vi "XY_plot_gnuplot.vi"(0 "Plot Array":cluster{dbl[], dbl[]}[](array[cluster])=[{[500.0, 500.0, 953.54, 215.0, 270.0, 320.0, 445.0, 525.0, 600.0, 675.0, 750.0, 825.0, 900.0, 960.0, 1010.0, 1060.0], [4.614524, 4.54365, 5.818368, 0.1374656, 0.6662545, 1.465458, 3.619824, 4.848976, 5.887329, 5.940571, 6.152151, 5.717487, 5.600293, 5.40069, 5.154843, 5.121789]}, {[100.0, 150.0, 215.0, 270.0, 320.0, 445.0, 525.0, 600.0, 675.0, 750.0, 825.0, 900.0, 960.0, 1010.0, 1060.0], [0.002314715, -0.00693192, 0.120417, 0.6880509, 1.519176, 3.513709, 5.065183, 6.116033, 6.096773, 5.938465, 5.593788, 5.5597, 5.387002, 5.304077, 4.887903]}] {"?" format="%.2f"; "?" format="%.2f"}, 1 "Job Directory":path=path "/G4_2_HD/Users/paulhayden/Documents/Projects/Westlakes_resolution") -> (2 "Saved Automatically?":bool, 3 "Tex Info String":string="set term epslatex\nset output \"Plot.eps\"\nset xlabel '$Distance~(m)$'\nset ylabel '$DF~(s/m^3)\\times10^6$'\nset samples 1000\nset pointsize 1.00\nset title '$B38~Centreline~Glc$' 0, 0\nset size 0.75,0.9\n\n#set key 450, -2.5833\n unset key\nset label 1 '~~~~~~~~~~~Angle~(deg)~=~0' at -100, -2.58\nset label 2 '~~~~~~~~~~~Height~(m)~=~5' at -100, -3.27\n set xrange [0 : 500] \n# set autoscale x \n set yrange [0.10000 : 7]\n# set autoscale y \n\nplot \"B38_Centreline_Glc.dat\" index 0 using 1:2 axes x1y1 title '$File=B38R~DDD.xls$' with points 1 1, \\\n\"B38_Centreline_Glc.dat\" index 1 using 1:2 axes x1y1 title '$File=B38R~DDD~1.xls$' with points 1 3", 4 "Plot data file":path)   [LabVIEW 2015]
uses:
  Gnuplot_Label.ctl
  gnuplotScriptComponents/gridlines.ctl
  gnuplotScriptComponents/legendAppearance.ctl
  gnuplotScriptComponents/legendProperties.ctl
  gnuplotScriptComponents/alignment.ctl
  gnuplotScriptComponents/at.ctl
  <vilib>/Analysis/baseanly.llb/Mean (DBL).vi
  Results_plotter_Global.vi
  <vilib>/Analysis/NI_AALBase.lvlib
  <vilib>/Analysis/NI_AALPro.lvlib
panel:
  in  "Current Fit Formula":string
  in  "Show Re-Run Gnuplot?":bool
  in  "Tab Control":T1(tab)
  in  "Plot Title":u16(ring) items=["Title String Only", "Stack::", "RunNum::", "WD::(deg)", "EBD::", "Stack:X:(mm ref TTC)", "User:Comments:", "Run:Messages:", "Exclude:Reason:", "X:Rel:(mm)", "Y:Rel:(mm)", "C:minusBG:(ppm)", "C:LatFit:Max(ppm)", "C:LatFit:SigmaY(mm)", "C:LatFit:Yo(mm)", "C:LatData:Max(ppm)", "Uref::(m/s)", "C:incBG:(ppm)", "C:Variance:(ppm^2)", "C:minusBG:(ppm)Err", "C:LatData:Max(ppm)Err", "BG:Conc:(ppm)", "BG:Variance:(ppm^2)", "BG:Conc:(ppm)Err", "FID:Num:", "FID:Calibration:Filename", "X:Trav:(mm)", "Y:Trav:(mm)", "Z (mm)::", "TrackedStack:Yat0deg:(mm)", "TrackedStack:Xat0deg:(mm)", "TrackedStack:Ycurrent:(mm)", "TrackedStack:Xcurrent:(mm)", "T::(C)", "P:Atm:(mbar)", "MFC:Enable:", "MFC24:Read:(%)", "MFC23:Read:(%)", "Date:of:Measurement", "Time:Measurement:Commenced", "Multi Run:Command:Filename", "Multi Run:Start Time:", "Multi Run:Row:Type", "Time:Stamp:(seconds)", "Original:Results:Filename", "Raw:Data:Filename", "EBD:Comments:", "EBD:Xdim:", "EBD:Ydim:", "EBD:Zdim:", "EBD:RunNum:", "EBD:X-Location:", "EBD:Y-Location:", "Number of Measurements"]
  in  "Plot Title":string
  in  "Added labels":i32[](listbox)
  in  "Show Labels?":bool
  in  "Summarise":u16(ring) items=["All Series", "EBD=0L\\times0W\\times0H @  0X, 0Y__Stack X (mm ref TTC)=Show All__", "EBD=80L\\times160W\\times80H @  -80X, 0Y__Stack X (mm ref TTC)=Show All__", "EBD=80L\\times160W\\times80H @  0X, 0Y__Stack X (mm ref TTC)=Show All__", "EBD=90L\\times180W\\times90H @  0X, 0Y__Stack X (mm ref TTC)=Show All__", "EBD=100L\\times200W\\times100H @  -100X, 0Y__Stack X (mm ref TTC)=Show All__"]
  in  "X Log?":bool
  in  "Y Log?":bool
  in  "Ymin Val":dbl
  in  "Ymin":bool=TRUE
  in  "Xmin Val":dbl
  in  "Xmin":bool=TRUE
  in  "Xmax Val":dbl
  in  "Xmax":bool=TRUE
  in  "Ymax Val":dbl
  in  "Ymax":bool=TRUE
  in  "Major Gridlines":T2
  in  "Minor Gridlines":T2
  out "Time format?":bool
  in  "precision":string
  out "Profile offset":dbl
  in  "Offset?":bool
  in  "Mode":T3
  in  "Separation":dbl=1.2
  in  "Fit Line Width":i32=2
  in  "Fit type":T4(ring)
  in  "Put Coeff\nin Results file":bool
  in  "Analysis":T5(ring)
  in  "Wavelength?":bool
  in  "Auto Zp":bool=TRUE
  in  "Fixed Zp":dbl format="%.2f"
  in  "Something about fit..!":bool
  in  "Fit Line Type":i32=2
  in  "Black and white?":bool
  in  "plot error bars?":bool
  in  "Plot style":u16[](array[ring])=[0, 0, 0, 0, 0, 0, 0, 0, 0, 0, 0] items=["points", "lines", "linespoints"]
  in  "Point Size":dbl=1.2 format="%.2f"
  in  "Graph Height":string="0.9"
  in  "Graph width":string="0.75"
  in  "Reverse order":bool
  in  "Appearance":T6
  in  "Show legend?":bool
  in  "Legend Position":u16(ring) items=["LabVIEW calculated", "top left", "top right", "bottom left", "bottom right", "below"]
  in  "Save data analysis file":bool
  out "Path":path
  in  "Filename Max length":i32=28
  out "With legend":i32=580
  out "No Legend":i32=397
  out "No of Series":i32=2
  out "X location":dbl=-100.0
  out "Y location":dbl=-2.583333333333333
  out "Delta y":dbl=0.6900000000000001
  out "Extra range":dbl
  out "Final Title":string="B38 Centreline Glc"
  out "XY Graph":cluster{dbl[], dbl[]}[](graph)=[{[215.0, 270.0, 320.0, 445.0, 500.0, 500.0, 525.0, 600.0, 675.0, 750.0, 825.0, 900.0, 953.54, 960.0, 1010.0, 1060.0], [0.1374656, 0.6662545, 1.465458, 3.619824, 4.614524, 4.54365, 4.848976, 5.887329, 5.940571, 6.152151, 5.717487, 5.600293, 5.818368, 5.40069, 5.154843, 5.121789]}, {[100.0, 150.0, 215.0, 270.0, 320.0, 445.0, 525.0, 600.0, 675.0, 750.0, 825.0, 900.0, 960.0, 1010.0, 1060.0], [0.002314715, -0.00693192, 0.120417, 0.6880509, 1.519176, 3.513709, 5.065183, 6.116033, 6.096773, 5.938465, 5.593788, 5.5597, 5.387002, 5.304077, 4.887903]}]
  # "Scales"
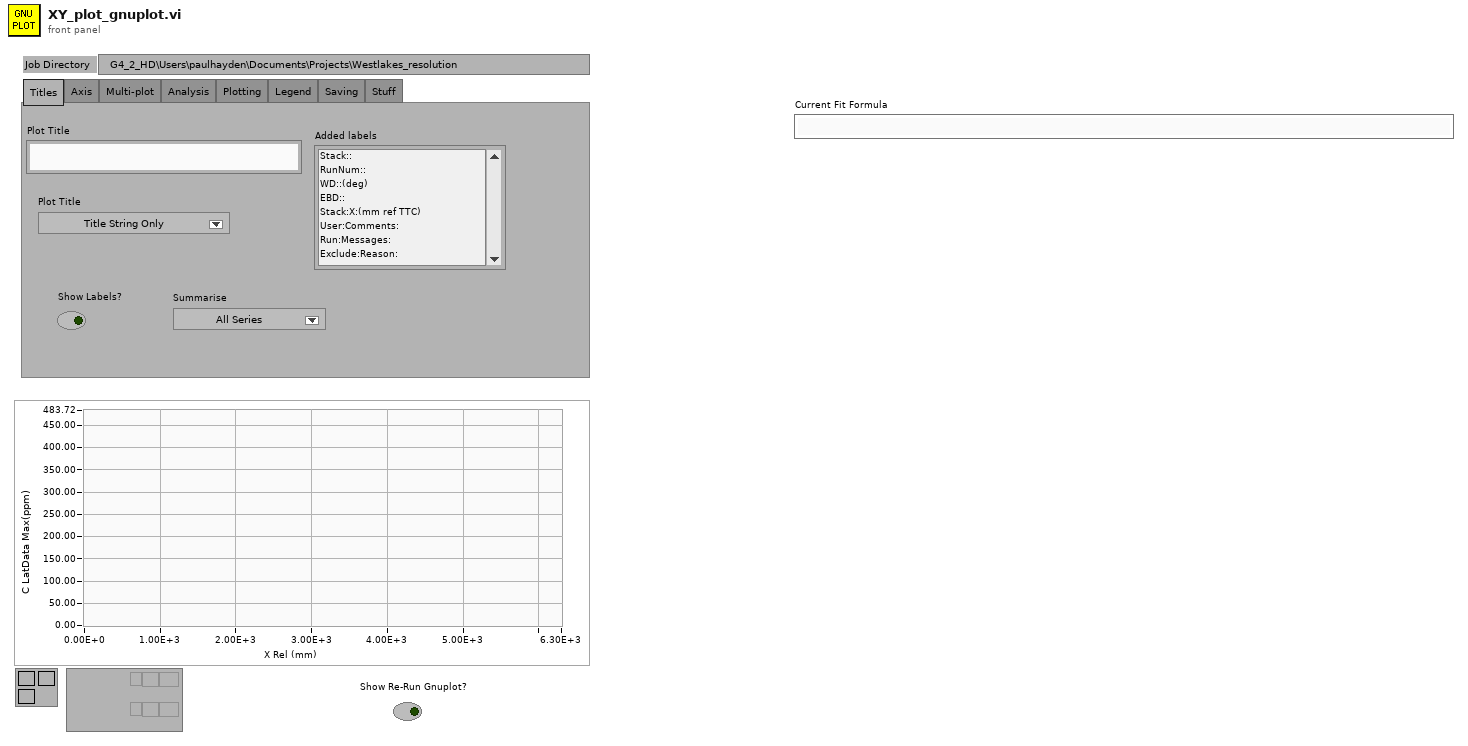
[diagram p1: front panel]
types:
  T1 = enum32{"Titles", "Axis", "Multi-plot", "Analysis", "Plotting", "Legend", "Saving", "Stuff"}
  T2 = typedef "gridlines.ctl" = enum16{"None", "X only", "Y only", "Both X and Y"}
  T3 = typedef "Gnuplot_Label.ctl" = enum16{"3 Labels per plot", "Only Center label", "Only Bottom Label"}
  T4 = enum16{"None", "Spline", "Linear", "2nd Poly", "3rd Poly", "4th Poly", "Gauss Lat", "Gauss vert", "Gauss Vert with 2 sig", "Guass glc"}
  T5 = enum16{"None", "% change", "Spectrum", "Norm Spec"}
  T6 = typedef "legendAppearance.ctl" = cluster{"layout":string, "text-sample order":string, "key order":string, "surroundingBox":string, "MaxRows":u32, "MaxCols":u32, "WidthAdjust":dbl}
  T7 = cluster{"Output":dbl[], "PercentageDifferenceArray":dbl[]}[]
  T8 = cluster{"Output":dbl[], "PercentageDifferenceArray":dbl[]}
  T9 = typedef "legendProperties.ctl" = cluster{"Appearance":T6, "Alignment":T10, "Location":string, "\"At\" location":T11}
  T10 = typedef "alignment.ctl" = cluster{"Horizontal":string, "Vertical":string}
  T11 = typedef "at.ctl" = cluster{"XcoordSys":string, "YcoordSys":string, "Xvalue":dbl, "Yvalue":dbl}
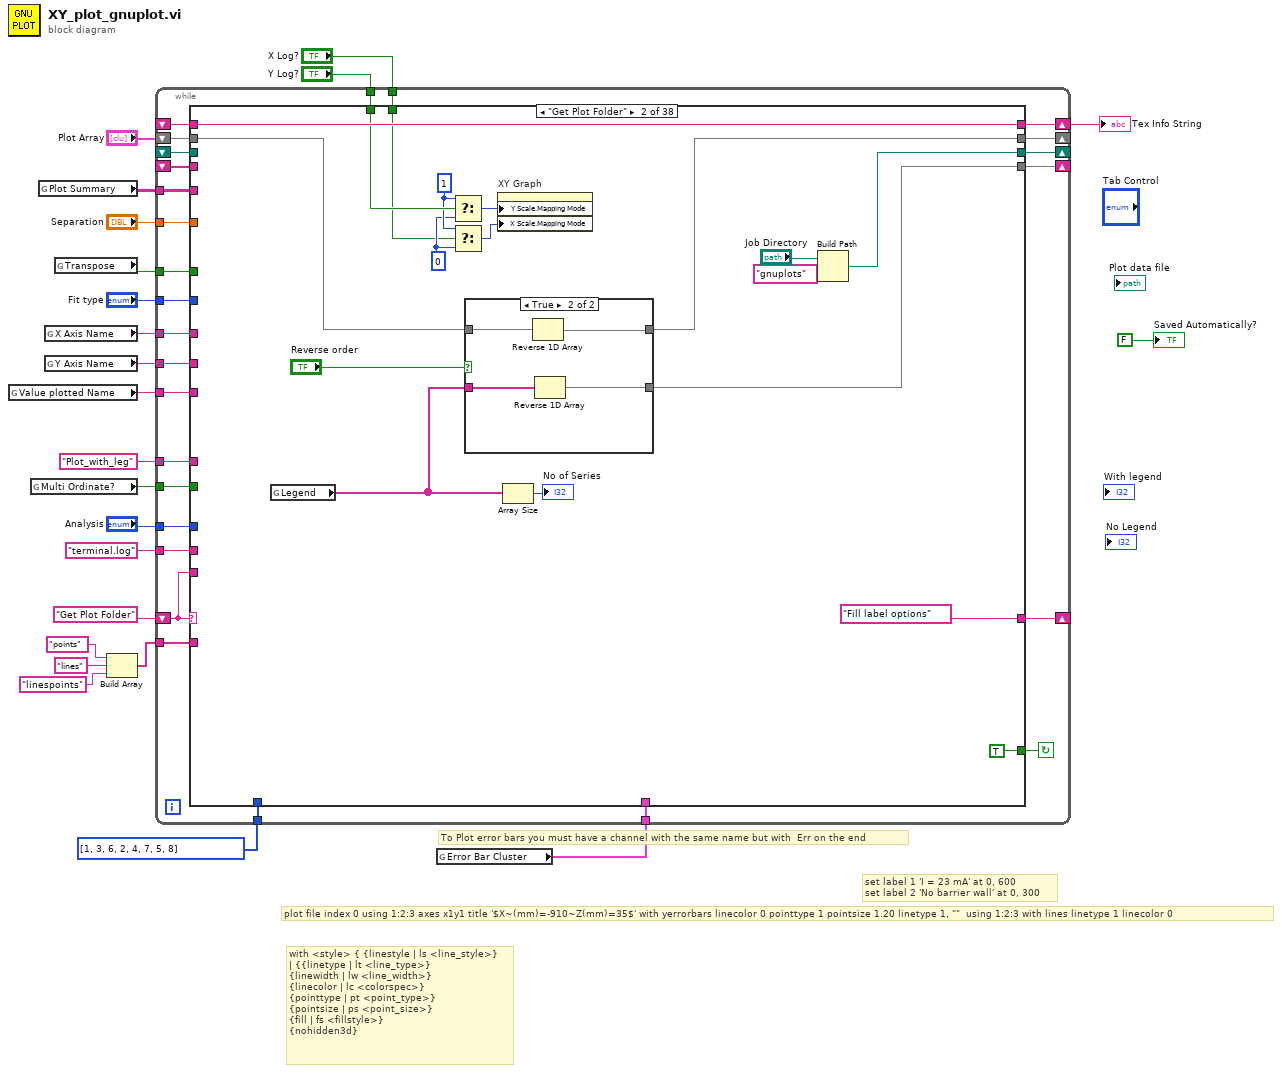
[diagram p0: block diagram]
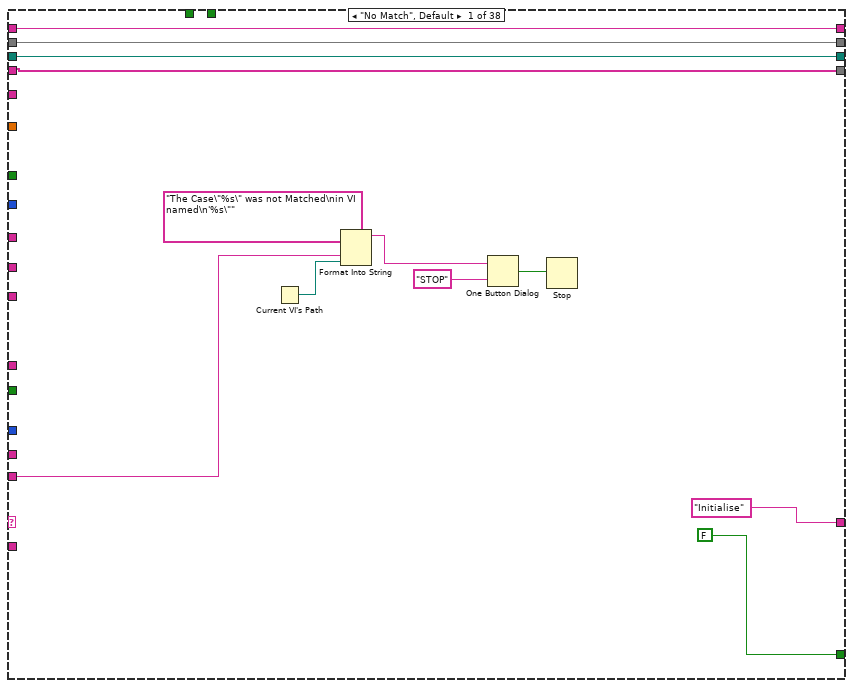
[diagram p2: hidden frame]
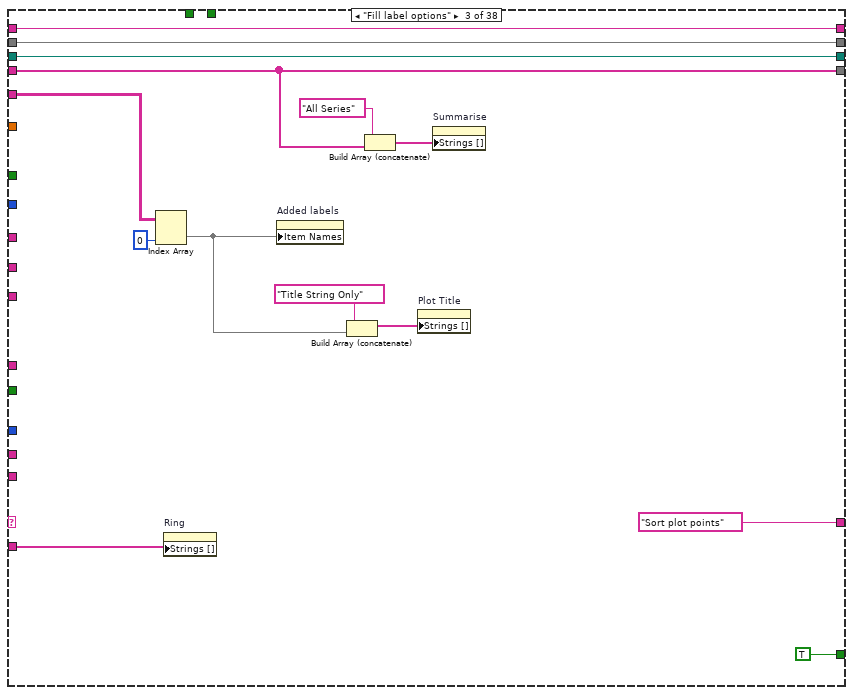
[diagram p4: hidden frame]
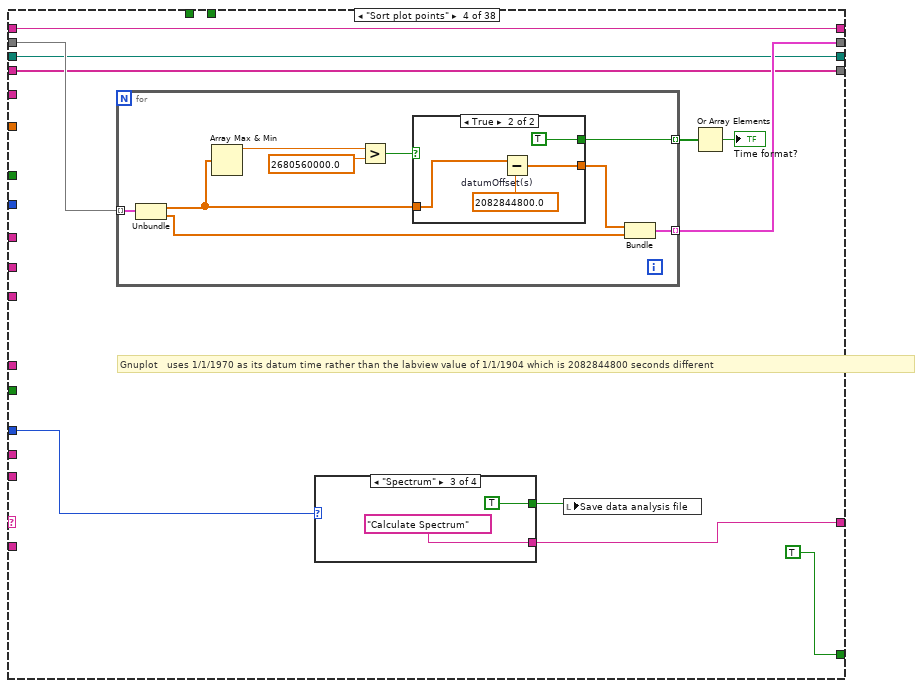
[diagram p5: hidden frame]
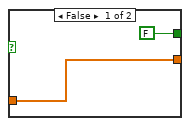
[diagram p6: hidden frame]
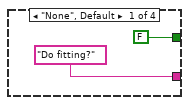
[diagram p7: hidden frame]
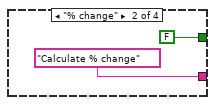
[diagram p8: hidden frame]
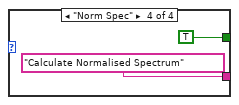
[diagram p9: hidden frame]
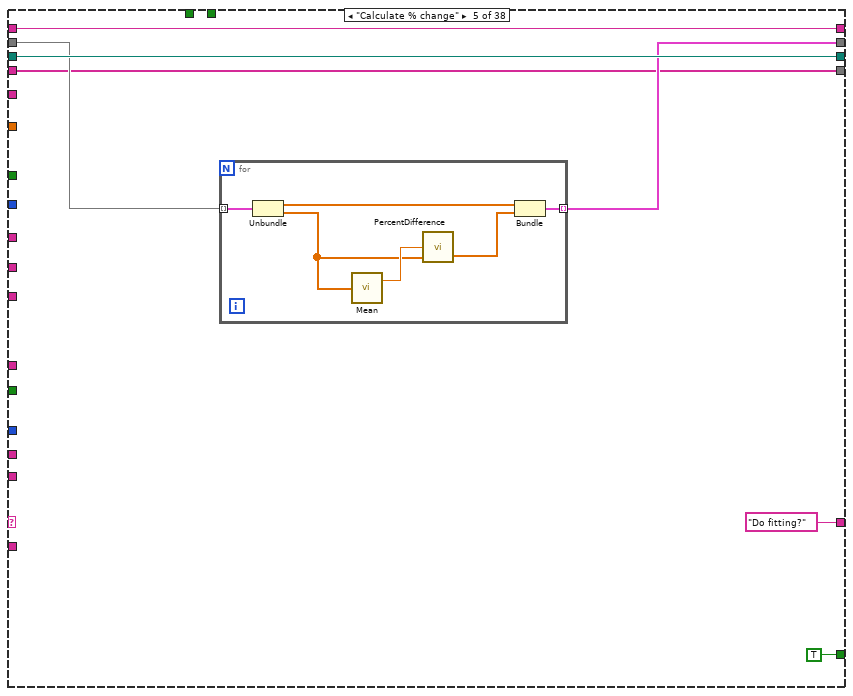
[diagram p10: hidden frame]
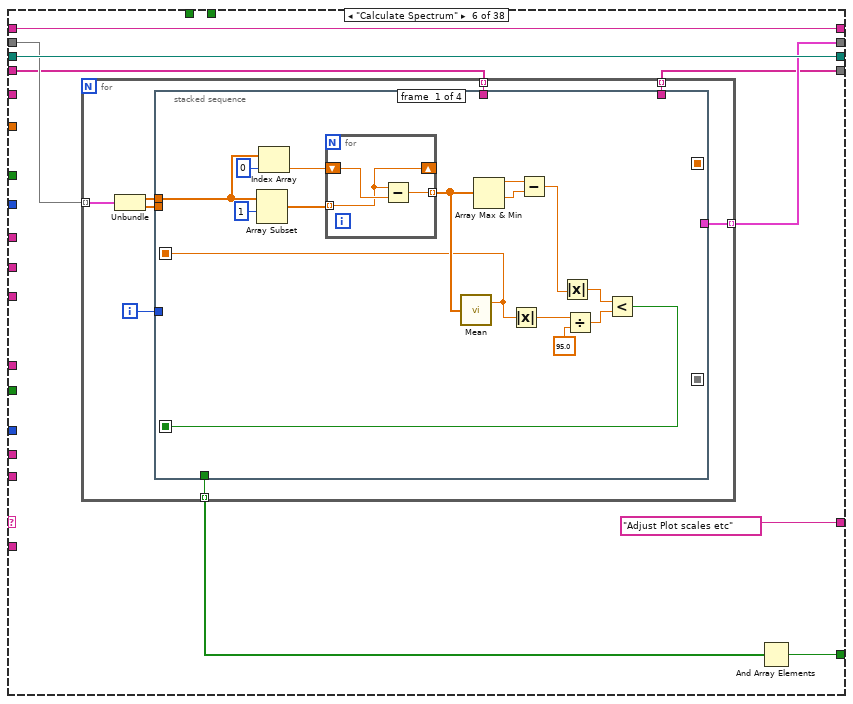
[diagram p11: hidden frame]
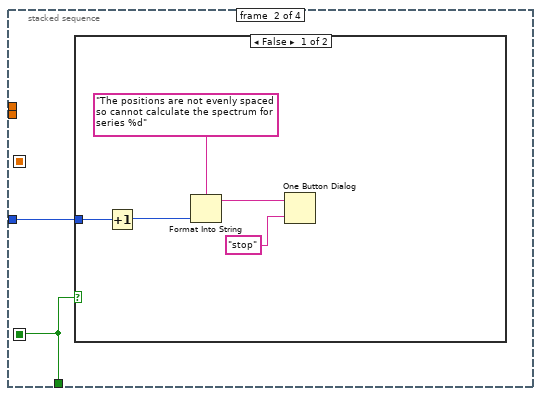
[diagram p12: hidden frame]
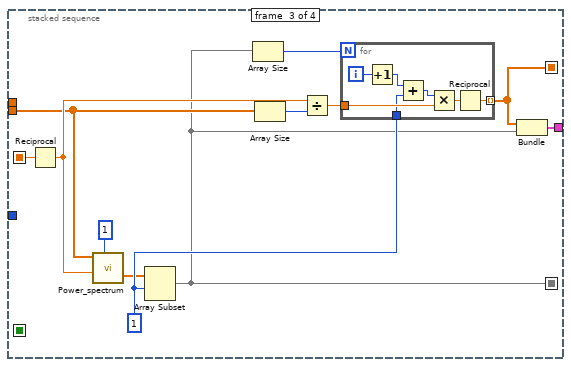
[diagram p14: hidden frame]
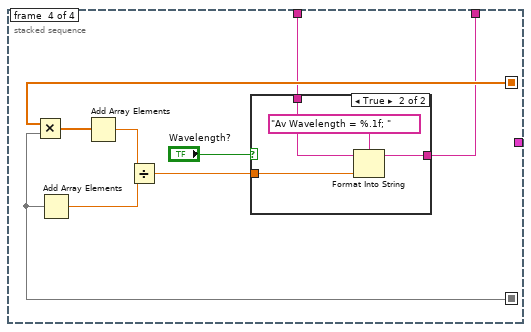
[diagram p15: hidden frame]
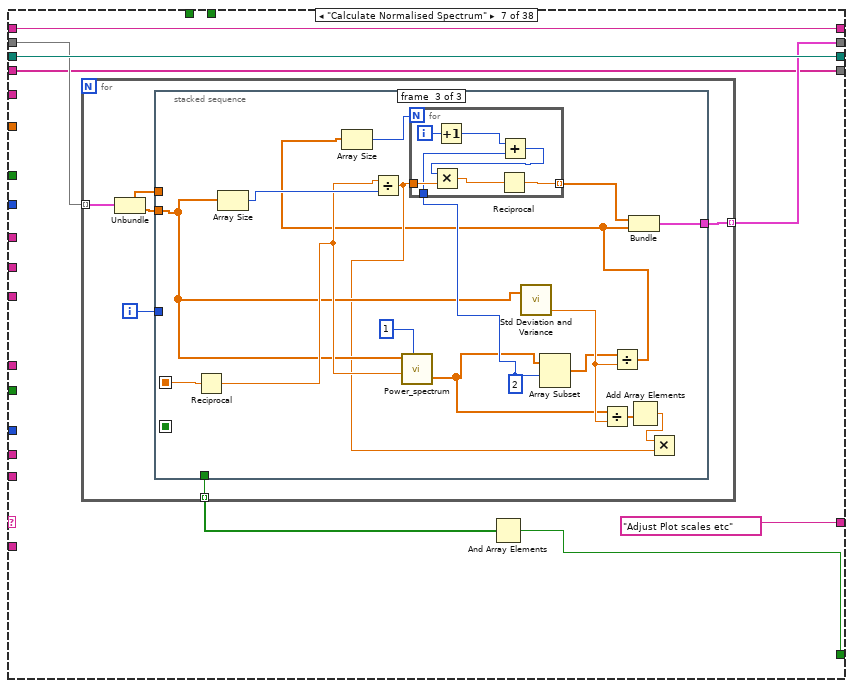
[diagram p17: hidden frame]
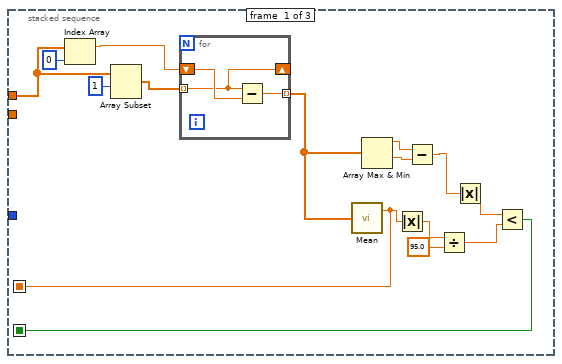
[diagram p18: hidden frame]
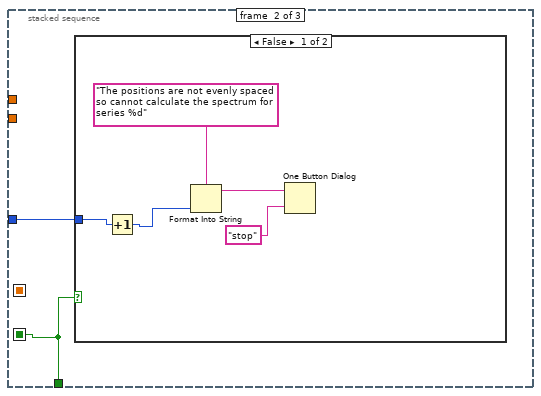
[diagram p19: hidden frame]
diagram:
  # "plot file index 0 using 1:2:3 axes x1y1 title '$X~(mm)=-910~Z(mm)=35$' with yerrorbars linecolor 0 pointtype 1 pointsize 1.20 linetype 1, \"\"  using 1:2:3 with lines linetype 1 linecolor 0"
  # "with <style> { {linestyle | ls <line_style>} \n| {{linetype | lt <line_type>} \n{linewidth | lw <line_width>} \n{linecolor | lc <colorspec>} \n{pointtype | pt <point_type>} \n{pointsize | ps <point_size>} \n{fill | fs <fillstyle>} \n{nohidden3d}"
  # "To Plot error bars you must have a channel with the same name but with  Err on the end"
  # "set label 1 'I = 23 mA' at 0, 600\nset label 2 'No barrier wall' at 0, 300"
  n1 = global read "Results_plotter_Global.vi" "Value plotted Name"() -> (w19:string)
  n2 = global read "Results_plotter_Global.vi" "Multi Ordinate?"() -> (w1:bool)
  n3 = global read "Results_plotter_Global.vi" "Plot Summary"() -> (w22:string[][])
  n4 = global read "Results_plotter_Global.vi" "X Axis Name"() -> (w21:string)
  n5 = global read "Results_plotter_Global.vi" "Y Axis Name"() -> (w20:string)
  n6 = global read "Results_plotter_Global.vi" "Transpose"() -> (w2:bool)
  n7 = Build Array("points", "lines", "linespoints") -> (w9:string[])
  n8 = global read "Results_plotter_Global.vi" "Error Bar Cluster"() -> (w4:cluster{string[]}[])
  n9 = while {
    shift-left: "Get Plot Folder" -> [w48]
    shift-right: [w49] -> _
    tunnel: w22 -> [w47]
    shift-right: [w46] -> _
    shift-left: _ -> [w45]
    tunnel: "Analysis" -> [w44]
    tunnel: w21 -> [w43]
    tunnel: w20 -> [w42]
    tunnel: w19 -> [w41]
    shift-right: [w39] -> _
    shift-left: "Plot Array" -> [w40]
    shift-right: [w37] -> w17
    shift-left: _ -> [w38]
    tunnel: "Plot_with_leg" ("name or relative path") -> [w36]
    tunnel: "Fit type" -> [w35]
    shift-right: [w34] -> _
    shift-left: _ -> [w33]
    tunnel: "terminal.log" -> [w32]
    tunnel: w9 -> [w31]
    tunnel: i32[] [1, 3, 6, 2, 4, 7, 5, 8] ("Plot style") -> [w30]
    tunnel: "Separation" -> [w29]
    tunnel: "Y Log?" -> [w28]
    tunnel: w4 -> [w27]
    tunnel: "X Log?" -> [w26]
    tunnel: w2 -> [w25]
    tunnel: w1 -> [w24]
    stop <- w50 continue-if-true
    n10 = case shown="\"Get Plot Folder\"" w48 {
      tunnel: [FALSE TRUE TRUE ("Top Level") TRUE TRUE w150 w223 TRUE TRUE TRUE ("Top Level") TRUE ("Top Level") TRUE ("Top Level") TRUE ("Top Level") TRUE ("Top Level") TRUE ("Top Level") TRUE ("Top Level") TRUE ("Top Level") TRUE ("Top Level") TRUE ("Top Level") TRUE ("Top Level") w674 w747 TRUE ("Top Level") TRUE ("Top Level") TRUE ("Top Level") TRUE ("Top Level") TRUE ("Top Level") TRUE ("Top Level") TRUE ("Top Level") TRUE ("Top Level") TRUE ("Top Level") TRUE ("Top Level") TRUE ("Top Level") TRUE ("Top Level") TRUE ("Top Level") w1578 FALSE ("Top Level") FALSE ("Top Level")] -> w50
      tunnel: ["Initialise" "Fill label options" "Sort plot points" w104 "Do fitting?" "Adjust Plot scales etc" "Adjust Plot scales etc" "Adjust Plot scales etc" "Add fitted line styles" "Adjust Plot scales etc" w381 "Fill Second legend" "Fill Second legend" "Fill Second legend" "Calculate plot max and min values" "Sort out plot title" w566 w636 "Create plot directory" w660 w673 w746 w890 "Edit Legend names" w1078 "Labels?" ("t") "Labels?" ("t") w1241 w1252 "Plot Command" "Write gnuplot file" ("t") "Execute shell script" ("t") "Has pdf been generated?" ("t") w1554 "Input Fit Coefficients into results file?" "Read Fit Coefficients" ("t") "End" ("t") "End" ("t")] -> w49
      tunnel: w48 -> [w57 _ _ _ _ _ _ _ _ _ _ _ _ _ _ _ _ _ _ _ _ _ _ _ _ _ _ _ _ _ _ _ _ _ _ _ _ _]
      tunnel: w47 -> [_ _ w100 _ _ _ _ _ _ _ _ _ _ _ _ _ w575 _ _ _ w672 w745 _ _ _ _ _ _ w1251 _ _ _ _ _ _ _ _ _]
      tunnel: [w54 w77 w94 w108 w139 w155 w229 w290 w305 w366 w391 w417 w426 w438 w465 w499 w568 w637 w648 w662 w675 w748 w902 w944 w1093 w1161 w1218 w1248 w1258 w1384 w1416 w1539 w1547 w1560 w1571 w1582 w1600 w1727] -> w46
      tunnel: w45 -> [w54 _ w94 w108 w139 w155 w229 w290 w305 w366 w391 w417 w426 w438 w461 w499 w567 w633 w649 w657 w675 w748 w902 w944 w1093 w1161 w1218 w1248 w1258 w1384 w1416 w1539 w1547 w1560 w1571 w1582 w1600 w1727]
      tunnel: w44 -> [_ _ _ w105 _ _ _ _ _ _ w382 _ _ w432 _ _ _ w624 _ _ w668 w740 w899 _ _ _ _ _ _ _ _ _ _ _ _ _ _ _]
      tunnel: w43 -> [_ _ _ _ _ _ _ _ w296 _ _ w413 w425 _ _ _ _ _ _ _ w671 w744 w897 _ _ _ _ _ _ _ _ _ _ _ _ _ _ _]
      tunnel: w42 -> [_ _ _ _ _ _ _ _ w295 _ _ w412 w424 w437 _ _ _ _ _ _ w670 w743 w898 _ _ _ _ _ _ _ _ _ _ _ _ _ _ _]
      tunnel: w41 -> [_ _ _ _ _ _ _ _ _ _ _ _ _ _ _ _ _ _ _ _ w667 _ _ _ _ _ _ _ _ _ _ _ _ _ _ _ w1588 _]
      tunnel: w40 -> [w53 w72 w95 w110 w138 w154 w228 w286 w301 w365 w380 w416 w423 w436 w464 w496 w581 w635 w652 w665 w666 w742 w903 w932 w1088 w1156 w1214 w1245 w1253 w1385 w1417 w1545 w1552 w1567 w1576 w1586 w1593 w1732]
      tunnel: [w53 w71 w95 w109 w137 w153 w227 w286 w294 w365 w380 w416 w423 w436 w464 w496 w581 w635 w652 w665 w666 w739 w903 w932 w1088 w1156 w1214 w1245 w1253 w1385 w1417 w1545 w1552 w1567 w1576 w1586 w1593 w1732] -> w39
      tunnel: w38 -> [w52 w76 w96 w107 w136 w152 w226 w289 w304 w363 w383 w415 w422 w435 w463 w500 w576 w634 w651 w664 w676 w749 _ w942 w1092 w1127 w1194 w1236 w1255 w1382 w1414 w1534 w1550 w1565 w1574 w1584 w1603 w1730]
      tunnel: [w52 w76 w96 w107 w136 w152 w226 w289 w304 w363 w383 w415 w422 w435 w463 w500 w576 w634 w651 w664 w676 w749 w893 w940 w1092 w1124 w1193 w1235 w1256 w1378 w1413 w1534 w1550 w1565 w1574 w1584 w1603 w1730] -> w37
      tunnel: w36 -> [_ _ _ _ _ _ _ _ _ _ _ _ _ _ _ _ _ _ _ _ _ _ _ _ _ _ _ _ _ _ _ _ _ _ _ _ _ _]
      tunnel: w35 -> [_ _ _ _ _ _ _ w287 w303 _ w385 _ _ _ _ _ _ _ _ _ _ _ w891 w946 _ _ _ _ _ w1351 w1410 _ _ _ _ w1581 w1596 _]
      tunnel: [w51 w70 w92 w106 w135 w148 w225 w288 w298 w362 w387 w414 w421 w434 w462 w498 w580 w632 w650 w663 w669 w741 w901 w947 w1094 w1160 w1217 w1247 w1257 w1372 w1415 w1540 w1551 w1566 w1575 w1585 w1604 w1731] -> w34
      tunnel: w33 -> [w51 _ w92 w106 w135 w149 w225 w288 w299 w362 w387 w414 w421 w434 w462 w498 w580 w632 w650 w663 w669 w741 w901 w947 w1095 w1160 w1217 w1247 w1257 w1372 w1415 w1540 w1551 w1566 w1575 w1585 w1604 w1731]
      tunnel: w32 -> [_ _ _ _ _ _ _ _ _ _ _ _ _ _ _ _ _ _ _ _ _ _ _ _ _ _ _ _ _ _ _ _ w1546 _ _ _ _ w1725]
      tunnel: w31 -> [_ _ w90 _ _ _ _ _ _ _ _ _ _ _ _ _ _ _ _ _ _ _ _ _ _ _ _ _ _ _ _ _ _ _ _ _ _ _]
      tunnel: w30 -> [_ _ _ _ _ _ _ _ _ _ _ _ _ _ _ _ _ _ _ _ _ _ _ _ _ _ _ _ _ _ w1408 w1536 _ _ _ _ _ _]
      tunnel: w29 -> [_ _ _ _ _ _ _ _ _ _ _ _ _ _ _ _ _ _ _ _ _ w738 _ _ w1087 _ _ _ _ w1369 _ _ _ _ _ _ _ _]
      tunnel: w28 -> [_ w69 _ _ _ _ _ _ _ _ _ _ _ _ _ _ _ _ _ _ _ _ _ _ _ w1140 w1205 _ w1250 w1366 _ _ _ _ _ _ _ _]
      tunnel: w27 -> [_ _ _ _ _ _ _ _ _ _ _ _ _ _ _ w469 _ _ _ _ _ w737 _ _ _ _ _ _ _ _ w1407 _ _ _ _ _ _ _]
      tunnel: w26 -> [_ w64 _ _ _ _ _ _ _ _ _ _ _ _ _ _ _ _ _ _ _ _ _ _ _ w1137 _ _ w1249 w1361 _ _ _ _ _ _ _ _]
      tunnel: w25 -> [_ _ _ _ _ _ _ _ _ _ _ _ _ _ _ w467 _ _ _ _ _ w736 _ w933 _ _ _ _ _ w1356 w1404 _ _ _ _ _ _ _]
      tunnel: w24 -> [_ _ _ _ _ _ _ _ _ _ _ _ _ _ _ _ _ _ _ _ _ _ _ _ _ _ _ _ _ _ _ _ _ _ _ _ _ _]
      frame "No Match", Default {
        n11 = Current VI's Path() -> (path=w56:path)
        n12 = Format Into String(format string="The Case\"%s\" was not Matched\nin VI named\n'%s\"" ("Format String"), w57, w56) -> (resulting string=w60:string)  [unwired: 2 in, 1 out]
        n13 = One Button Dialog(message=w60, button name ("OK")="STOP") -> (true=w58:bool)
        n14 = Stop(stop? (T)=w58) -> ()
      }
      frame "Get Plot Folder" {
        w65 = u8 0 ("f")
        w66 = u8 1 ("Y Scale.Mapping Mode")
        n15 = global read "Results_plotter_Global.vi" "Legend"() -> (w63:string[])
        n16 = Select(t=w66, s=w69, f=w65) -> (s? t:f=w68:u8)
        n17 = Select(t=w66, s=w64, f=w65) -> (s? t:f=w67:u8)
        n18 = case shown="True" "Reverse order" {
          tunnel: w72 -> [w82 w86]
          tunnel: [w82 w85] -> w71
          tunnel: w63 -> [w81 w84]
          tunnel: [w81 w83] -> w70
          frame False {
          }
          frame True {
            n19 = Reverse 1D Array(array=w86) -> (reversed array=w85:T7)
            n20 = Reverse 1D Array(array=w84) -> (reversed array=w83:string[])
          }
        }
        n21 = property on="XY Graph" class="XYGraph (strict)"("Y Scale.Mapping Mode"=w68, "X Scale.Mapping Mode"=w67) -> ()  [unwired: 2 in, 2 out]
        n22 = Array Size(array=w63) -> (size(s)=→"No of Series":i32)
        n23 = Build Path(base path="Job Directory", name or relative path="gnuplots") -> (appended path=w77:path)
      }
      frame "Fill label options" {
        n24 = Index Array(array=w100, index (col)=0 ("disabled index (col)")) -> (element=w88:string[])  [unwired: 1 in]
        n25 = property on="Ring" class="Ring (strict)"("Strings []"=w90) -> ()  [unwired: 2 in, 2 out]
        n26 = property on="Added labels" class="LstBox (strict)"("Item Names"=w88) -> ()  [unwired: 2 in, 2 out]
        n27 = Build Array (concatenate)("Title String Only", w88) -> (w87:string[])
        n28 = Build Array (concatenate)("All Series", w92) -> (w93:string[])
        n29 = property on="Plot Title" class="Ring (strict)"("Strings []"=w87) -> ()  [unwired: 2 in, 2 out]
        n30 = property on="Summarise" class="Ring (strict)"("Strings []"=w93) -> ()  [unwired: 2 in, 2 out]
      }
      frame "Sort plot points" {
        # "Gnuplot   uses 1/1/1970 as its datum time rather than the labview value of 1/1/1904 which is 2082844800 seconds different"
        n31 = for {
          tunnel: w110 -> [w119] mode=indexing
          tunnel: [w120] -> w109 mode=indexing
          tunnel: [w112] -> w102 mode=indexing
          n32 = Unbundle(w119) -> ("Output"=w115:dbl[], "PercentageDifferenceArray"=w116:dbl[])
          n33 = Array Max & Min(array=w115) -> (max value=w118:dbl)  [unwired: 3 out]
          n34 = Greater?(x=w118, y=2680560000.0) -> (0:w113:bool)
          n35 = case shown="True" w113 {
            tunnel: w115 -> [w122 w126]
            tunnel: [w122 w124] -> w114
            tunnel: [FALSE TRUE] -> w112
            frame False {
            }
            frame True {
              w125 = 2082844800.0  # datumOffset(s)
              n36 = Subtract(x=w126, y=w125) -> (x-y=w124:dbl[])
            }
          }
          n37 = Bundle("Output"=w114, "PercentageDifferenceArray"=w116) -> (w120:T8)  [unwired: 1 out]
        }
        n38 = case shown="\"Spectrum\"" w105 {
          tunnel: ["Do fitting?" "Calculate % change" "Calculate Spectrum" "Calculate Normalised Spectrum"] -> w104
          tunnel: [FALSE ("Save data analysis file") FALSE ("Save data analysis file") TRUE ("Save data analysis file") TRUE ("Save data analysis file")] -> w103
          frame "None", Default {
          }
          frame "% change" {
          }
          frame "Spectrum" {
          }
          frame "Norm Spec" {
          }
        }
        n39 = local write "Save data analysis file"(w103) -> ()
        n40 = Or Array Elements(Boolean array=w102) -> (logical OR=→"Time format?":bool)
      }
      frame "Calculate % change" {
        n41 = for {
          tunnel: w138 -> [w147] mode=indexing
          tunnel: [w145] -> w137 mode=indexing
          n42 = Unbundle(w147) -> ("Output"=w146:dbl[], "PercentageDifferenceArray"=w143:dbl[])
          n43 = call-poly <vilib>:"Mean.vi"("X"=w143) -> ("mean"=w144:dbl)  [unwired: 1 out]
          n44 = call "PercentDifference.vi"("CompareeArray"=w143, "Basis"=w144) -> ("PercentageDifferenceArray"=w142:dbl[])  [unwired: 1 in, 1 out]
          n45 = Bundle("Output"=w146, "PercentageDifferenceArray"=w142) -> (w145:T8)  [unwired: 1 out]
        }
      }
      frame "Calculate Spectrum" {
        n46 = for {
          tunnel: w154 -> [w163] mode=indexing
          tunnel: [w164] -> w153 mode=indexing
          tunnel: [w159] -> w151 mode=indexing
          tunnel: w149 -> [w158] mode=indexing
          tunnel: [w157] -> w148 mode=indexing
          i -> [w160]
          n47 = Unbundle(w163) -> ("Output"=w161:dbl[], "PercentageDifferenceArray"=w162:dbl[])
          n48 = stacked-sequence {
            seq-local: [w166 _ _ _] -> [_ _ w196 _]
            seq-local: [w165 _ _ _] -> [_ w183 _ _]
            seq-local: [_ _ w191 _] -> [_ _ _ w216]
            seq-local: [_ _ w190 _] -> [_ _ _ w217]
            tunnel: [_ _ w201 _] -> w164
            tunnel: w162 -> [_ _ w194 _]
            tunnel: w161 -> [w177 _ _ _]
            tunnel: w160 -> [_ w184 _ _]
            tunnel: [_ w183 _ _] -> w159
            tunnel: w158 -> [_ _ _ w212]
            tunnel: [_ _ _ w210] -> w157
            frame #0 {
              n49 = Array Subset(array=w177, index=1) -> (w175:dbl[])  [unwired: 1 in]
              n50 = Index Array(array=w177, index=0) -> (element=w176:dbl)
              n51 = for {
                shift-right: [w181] -> _
                shift-left: w176 -> [w182]
                tunnel: w175 -> [w181] mode=indexing
                tunnel: [w180] -> w172 mode=indexing
                n52 = Subtract(x=w181, y=w182) -> (x-y=w180:dbl)
              }
              n53 = call-poly <vilib>:"Mean.vi"("X"=w172) -> ("mean"=w166:dbl)  [unwired: 1 out]
              n54 = Array Max & Min(array=w172) -> (max value=w174:dbl, min value=w173:dbl)  [unwired: 2 out]
              n55 = Absolute Value(x=w166) -> (abs(x)=w169:dbl)
              n56 = Subtract(x=w174, y=w173) -> (x-y=w171:dbl)
              n57 = Absolute Value(x=w171) -> (abs(x)=w170:dbl)
              n58 = Divide(x=w169, y=95.0) -> (x/y=w167:dbl)
              n59 = Less?(x=w170, y=w167) -> (x < y?=w165:bool)
            }
            frame #1 {
              n60 = case shown="False" w183 {
                tunnel: w184 -> [w189 _]
                frame False {
                  n61 = Increment(x=w189) -> (x+1=w188:i32)
                  n62 = Format Into String(format string="The positions are not evenly spaced so cannot calculate the spectrum for series %d", w188) -> (resulting string=w186:string)  [unwired: 2 in, 1 out]
                  n63 = One Button Dialog(message=w186, button name ("OK")="stop") -> ()  [unwired: 1 out]
                }
                frame True {
                }
              }
            }
            frame #2 {
              w197 = 1 ("index")
              n64 = Reciprocal(x=w196) -> (1/x=w195:dbl)
              n65 = call "Power_spectrum.vi"("U"=w194, "Sampling frequency"=w195, "Block No"=1) -> ("Spectrum output array"=w193:dbl[])  [unwired: 1 in, 2 out]
              n66 = Array Subset(array=w193, index=w197) -> (w190:dbl[])  [unwired: 1 in]
              n67 = Array Size(array=w190) -> (size(s)=w200:i32)
              n68 = Array Size(array=w194) -> (size(s)=w198:i32)
              n69 = Divide(x=w195, y=w198) -> (x/y=w192:dbl)
              n70 = for {
                N: w200 -> [_]
                tunnel: [w205] -> w191 mode=indexing
                tunnel: w192 -> [w207]
                tunnel: w197 -> [w203]
                i -> [w208]
                n71 = Increment(x=w208) -> (x+1=w204:i32)
                n72 = Add(x=w204, y=w203) -> (x+y=w202:i32)
                n73 = Multiply(x=w202, y=w207) -> (x*y=w206:dbl)
                n74 = Reciprocal(x=w206) -> (1/x=w205:dbl)
              }
              n75 = Bundle(w191, w190) -> (w201:cluster{dbl[], dbl[]})  [unwired: 1 out]
            }
            frame #3 {
              n76 = Multiply(x=w216, y=w217) -> (x*y=w215:dbl[])
              n77 = Add Array Elements(numeric array=w217) -> (sum=w213:dbl)
              n78 = Add Array Elements(numeric array=w215) -> (sum=w214:dbl)
              n79 = Divide(x=w214, y=w213) -> (x/y=w211:dbl)
              n80 = case shown="True" "Wavelength?" {
                tunnel: w212 -> [w218 w222]
                tunnel: w211 -> [_ w221]
                tunnel: [w218 w219] -> w210
                frame False {
                }
                frame True {
                  n81 = Format Into String(format string="Av Wavelength = %.1f; ", initial string=w222, w221) -> (resulting string=w219:string)  [unwired: 1 in, 1 out]
                }
              }
            }
          }
        }
        n82 = And Array Elements(Boolean array=w151) -> (logical AND=w150:bool)
      }
      frame "Calculate Normalised Spectrum" {
        n83 = for {
          tunnel: w228 -> [w235] mode=indexing
          tunnel: [w236] -> w227 mode=indexing
          tunnel: [w231] -> w224 mode=indexing
          i -> [w232]
          n84 = Unbundle(w235) -> ("Output"=w233:dbl[], "PercentageDifferenceArray"=w234:dbl[])
          n85 = stacked-sequence {
            seq-local: [w238 _ _] -> [_ _ w271]
            seq-local: [w237 _ _] -> [_ w255 _]
            tunnel: [_ _ w277] -> w236
            tunnel: w234 -> [_ _ w269]
            tunnel: w233 -> [w249 _ _]
            tunnel: w232 -> [_ w256 _]
            tunnel: [_ w255 _] -> w231
            frame #0 {
              n86 = Index Array(array=w249, index=0) -> (element=w248:dbl)
              n87 = Array Subset(array=w249, index=1) -> (w247:dbl[])  [unwired: 1 in]
              n88 = for {
                shift-right: [w253] -> _
                shift-left: w248 -> [w254]
                tunnel: w247 -> [w253] mode=indexing
                tunnel: [w252] -> w244 mode=indexing
                n89 = Subtract(x=w253, y=w254) -> (x-y=w252:dbl)
              }
              n90 = call-poly <vilib>:"Mean.vi"("X"=w244) -> ("mean"=w238:dbl)  [unwired: 1 out]
              n91 = Array Max & Min(array=w244) -> (max value=w246:dbl, min value=w245:dbl)  [unwired: 2 out]
              n92 = Absolute Value(x=w238) -> (abs(x)=w241:dbl)
              n93 = Subtract(x=w246, y=w245) -> (x-y=w243:dbl)
              n94 = Divide(x=w241, y=95.0) -> (x/y=w239:dbl)
              n95 = Absolute Value(x=w243) -> (abs(x)=w242:dbl)
              n96 = Less?(x=w242, y=w239) -> (x < y?=w237:bool)
            }
            frame #1 {
              n97 = case shown="False" w255 {
                tunnel: w256 -> [w261 _]
                frame False {
                  n98 = Increment(x=w261) -> (x+1=w260:i32)
                  n99 = Format Into String(format string="The positions are not evenly spaced so cannot calculate the spectrum for series %d", w260) -> (resulting string=w258:string)  [unwired: 2 in, 1 out]
                  n100 = One Button Dialog(message=w258, button name ("OK")="stop") -> ()  [unwired: 1 out]
                }
                frame True {
                }
              }
            }
            frame #2 {
              w272 = 2 ("index")
              n101 = Reciprocal(x=w271) -> (1/x=w270:dbl)
              n102 = Array Size(array=w269) -> (size(s)=w273:i32)
              n103 = Divide(x=w270, y=w273) -> (x/y=w264:dbl)
              n104 = call "Power_spectrum.vi"("U"=w269, "Sampling frequency"=w270, "Block No"=1) -> ("Spectrum output array"=w267:dbl[])  [unwired: 1 in, 2 out]
              n105 = call <vilib>:"Std Deviation and Variance.vi"("X"=w269) -> ("variance"=w268:dbl)  [unwired: 1 in, 2 out]
              n106 = Array Subset(array=w267, index=w272) -> (w263:dbl[])  [unwired: 1 in]
              n107 = Divide(x=w267, y=w268) -> (x/y=w266:dbl[])
              n108 = Divide(x=w263, y=w268) -> (x/y=w262:dbl[])
              n109 = Array Size(array=w262) -> (size(s)=w276:i32)
              n110 = for {
                N: w276 -> [_]
                tunnel: [w281] -> w275 mode=indexing
                tunnel: w264 -> [w283]
                tunnel: w272 -> [w279]
                i -> [w284]
                n111 = Increment(x=w284) -> (x+1=w280:i32)
                n112 = Add(x=w280, y=w279) -> (x+y=w278:i32)
                n113 = Multiply(x=w278, y=w283) -> (x*y=w282:dbl)
                n114 = Reciprocal(x=w282) -> (1/x=w281:dbl)
              }
              n115 = Bundle(w275, w262) -> (w277:cluster{dbl[], dbl[]})  [unwired: 1 out]
              n116 = Add Array Elements(numeric array=w266) -> (sum=w265:dbl)
              n117 = Multiply(x=w265, y=w264) -> ()  [unwired: 1 out]
            }
          }
        }
        n118 = And Array Elements(Boolean array=w224) -> (logical AND=w223:bool)
      }
      frame "Do fitting?" {
        n119 = case shown="\"Linear\", Default" w287 {
          tunnel: ["Adjust Plot scales etc" "Poly fit to data"] -> _
          frame "None" {
          }
          frame "Linear", Default {
          }
        }
      }
      frame "Poly fit to data" {
        n120 = case shown="\"None\", Default" w303 {
          tunnel: [0 ("polynomial order") 1 ("polynomial order") 2 ("polynomial order") 3 ("polynomial order") 4 ("polynomial order")] -> w302
          frame "None", Default {
          }
          frame "Linear" {
          }
          frame "2nd Poly" {
          }
          frame "3rd Poly" {
          }
          frame "4th Poly" {
          }
        }
        n121 = for {
          tunnel: w301 -> [w325] mode=indexing
          tunnel: [w326] -> w300 mode=indexing
          tunnel: w302 -> [w324]
          tunnel: [w319] -> w297 mode=indexing
          tunnel: w296 -> [w318]
          tunnel: w295 -> [w317]
          w323 = 8  # Enhancement factor
          n122 = Unbundle(w325) -> ("Output"=w316:dbl[], "PercentageDifferenceArray"=w315:dbl[])
          n123 = call <vilib>:"General Polynomial Fit.vi"("Y"=w315, "polynomial order"=w324, "X"=w316) -> ("Polynomial Coefficients"=w313:dbl[])  [unwired: 9 in, 3 out]
          n124 = case shown="False" "Something about fit..!" {
            tunnel: [w329 w344] -> w320
            tunnel: [w340 w345] -> w319
            tunnel: w318 -> [w342 _]
            tunnel: w317 -> [w341 _]
            tunnel: w316 -> [w337 _]
            tunnel: w315 -> [w334 _]
            tunnel: w313 -> [_ w344]
            frame False {
              w336 = 0.99 ("Voltage")
              n125 = Build Array (concatenate)(nan ("Voltage"), w334) -> (w338:dbl[])
              n126 = Build Array (concatenate)(w336, w337) -> (w339:dbl[])
              n127 = call "Curve_Fit_ph.vi"("Values In"=w338, "No of points to fit (3)"=4, "Positions"=w339) -> ("Values Out"=w333:dbl[], "Polynomial Fit Coefficients"=w329:dbl[])  [unwired: 1 in]
              n128 = Index Array(array=w333, index=0) -> (element=w331:dbl)
              n129 = call "Number_2_string.vi"("precision"="2", "number"=w331) -> ("String"=w327:string)
              n130 = Format Into String(format string="When %s=%.2f ; %s=%s", w342, w336, w341, w327) -> (resulting string=w340:string)  [unwired: 2 in, 1 out]
            }
            frame True {
              n131 = for {
                shift-right: [w347] -> w345
                shift-left: "" -> [w348]
                tunnel: w344 -> [w351] mode=indexing
                i -> [w352]
                n132 = call "Number_2_string.vi"("number"=w351) -> ("String"=w349:string)  [unwired: 1 in]
                n133 = case shown="0, Default" w352 {
                  tunnel: [w353] -> w350
                  tunnel: w349 -> [w355]
                  frame 0, Default {
                    n134 = Concatenate Strings(w355, " ") -> (w353:string)
                  }
                }
                n135 = Concatenate Strings(w348, w350) -> (w347:string)
              }
            }
          }
          n136 = call "Enhance_No_of_points.vi"("Enhancement factor"=w323, "Input"=w316) -> ("Output"=w322:dbl[])  [unwired: 3 out]
          n137 = for {
            tunnel: w320 -> [w358]
            tunnel: w322 -> [w357] mode=indexing
            tunnel: [w356] -> w321 mode=indexing
            n138 = call "Polynomial_convert.vi"("Calib constants"=w358, "Voltage"=w357) -> ("Eng Values"=w356:dbl)  [unwired: 4 out]
          }
          n139 = Bundle("Output"=w322, w321) -> (w326:cluster{"Output":dbl[], dbl[]})  [unwired: 1 out]
        }
        n140 = Build Array (concatenate)(w299, w297) -> (w298:string[])
        n141 = Build Array (concatenate)(w301, w300) -> (w294:T7)
        n142 = local write "XY Graph"(w294) -> ()
      }
      frame "Add fitted line styles" {
        n143 = local read "No of Series"() -> (w359:i32)
        n144 = Array Subset(array=w362, index=w359) -> (w361:string[])  [unwired: 1 in]
        n145 = for {
          tunnel: w361 -> [w370] mode=indexing
          tunnel: u8 2 ("Plot.Plot Interpolation") -> [w376]
          tunnel: w359 -> [w372]
          i -> [w373]
          w378 = u32 0
          n146 = Concatenate Strings(w370, "  " ("string")) -> (w368:string)
          n147 = Add(x=w372, y=w373) -> (x+y=w371:i32)
          n148 = Quotient & Remainder(x=w373, y=4) -> (x-y*floor(x/y)=w374:i32)  [unwired: 1 out]
          n149 = property on="XY Graph" class="XYGraph (strict)"("Active Plot"=w371, "Plot.Plot Name"=w368, "Plot.Fill/Point Color"=w378, "Plot.Plot Color"=w378, "Plot.Point Style"=u8 0, "Plot.Line Style"=w374, "Plot.Plot Interpolation"=w376) -> ()  [unwired: 2 in, 2 out]
        }
      }
      frame "Adjust Plot scales etc" {
        w379 = u8[] [6, 1, 11, 2, 5, 13, 15, 10, 12, 14]  # pointStyles
        n150 = Greater Than 0?(x=w385) -> (x > 0?=w384:bool)
        n151 = Array Size(array=w387) -> (size(s)=w392:i32)
        n152 = local read "No of Series"() -> (w386:i32)
        n153 = property on="XY Graph" class="XYGraph (strict)"("Legend:Plots Shown"=w392) -> ()  [unwired: 2 in, 2 out]
        n154 = case shown="\"None\", Default" w382 {
          tunnel: ["Adjust plot scales2" "Show percentage change" ("t") "Set spectra axis" ("t") "Set spectra axis" ("t")] -> w381
          frame "None", Default {
          }
          frame "% change" {
          }
          frame "Spectrum" {
          }
          frame "Norm Spec" {
          }
        }
        n155 = Select(t=u8 2 ("Plot.Plot Interpolation"), s=w384, f=u8 0 ("Plot.Plot Interpolation")) -> (s? t:f=w388:u8)
        n156 = for {
          N: w386 -> [_]
          tunnel: w387 -> [w406] mode=indexing
          tunnel: w379 -> [w410]
          tunnel: w388 -> [w399]
          i -> [w409]
          w411 = u32 0
          n157 = String Length(string=w406) -> (length=w402:i32)
          n158 = Subtract(x=w402, y=2) -> (x-y=w400:i32)
          n159 = String Subset(string=w406, offset (0)=0, length (rest)=w400) -> (substring=w405:string)
          n160 = Concatenate Strings(w405, "  " ("string")) -> (w403:string)
          n161 = Index Array(array=w410, index=w409) -> (element=w408:u8)
          n162 = property on="XY Graph" class="XYGraph (strict)"("Active Plot"=w409, "Plot.Plot Name"=w403, "Plot.Fill/Point Color"=w411, "Plot.Plot Color"=w411, "Plot.Point Style"=w408, "Plot.Line Style"=u8 0, "Plot.Plot Interpolation"=w399) -> ()  [unwired: 2 in, 2 out]
        }
        "XY Graph" <- w380
      }
      frame "Adjust plot scales2" {
        n163 = property on="XY Graph" class="XYGraph (strict)"("X Scale.Name Label.Text"=w413, "Y Scale.Name Label.Text"=w412, "Cursor.Visible"=FALSE) -> ()  [unwired: 2 in, 2 out]
      }
      frame "Show percentage change" {
        n164 = Concatenate Strings(w424, " % Change" ("string")) -> (w427:string)
        n165 = property on="XY Graph" class="XYGraph (strict)"("X Scale.Name Label.Text"=w425, "Y Scale.Name Label.Text"=w427, "Cursor.Visible"=FALSE) -> ()  [unwired: 2 in, 2 out]
      }
      frame "Set spectra axis" {
        n166 = case shown="\"Spectrum\", Default" w432 {
          tunnel: [" Spectral Energy" ("string") " Normalised Spectral Energy" ("string")] -> w440
          frame "Spectrum", Default {
          }
          frame "Norm Spec" {
          }
        }
        n167 = Concatenate Strings(w437, w440) -> (w439:string)
        n168 = property on="XY Graph" class="XYGraph (strict)"("X Scale.Name Label.Text"="Wavelength [mm]", "Y Scale.Name Label.Text"=w439, "Cursor.Visible"=FALSE) -> ()  [unwired: 2 in, 2 out]
      }
      frame "Fill Second legend" {
        n169 = global read "Results_plotter_Global.vi" "Current Data Filenames"() -> (w450:string)
        n170 = call "Fast_string_Replace.vi"("Replace match with:"="_", "Input String"=w450, "regular expression"="[/]") -> ("Output String"=w454:string)  [unwired: 2 out]
        n171 = call "Fast_string_Replace.vi"("Replace match with:"="_", "Input String"=w454, "regular expression"="__") -> ("Output String"=w451:string)  [unwired: 2 out]
        n172 = call "Fast_string_Replace.vi"("Replace match with:"="", "Input String"=w451, "regular expression"=" ") -> ("Output String"=w449:string)  [unwired: 2 out]
        n173 = String Subset(string=w449, offset (0)=0, length (rest)=30 ("length (rest)")) -> (substring=w448:string)
        n174 = Build Path(base path=w461, name or relative path=w448) -> (appended path=w465:path)
      }
      frame "Calculate plot max and min values" {
        n175 = local read "plot error bars?"() -> (w468:bool)
        n176 = for {
          tunnel: w496 -> [w524] mode=indexing
          shift-right: [w521] -> w492
          shift-left: _ -> [w517]
          shift-right: [w520] -> w493
          shift-left: _ -> [w516]
          shift-right: [w519] -> w487
          shift-left: _ -> [w515]
          shift-right: [w518] -> w486
          shift-left: _ -> [w514]
          tunnel: w469 -> [w512]
          tunnel: w468 -> [w513]
          tunnel: w467 -> [w510]
          i -> [w511]
          n177 = Unbundle(w524) -> ("Output"=w523:dbl[], "PercentageDifferenceArray"=w522:dbl[])
          n178 = case shown="True" w513 {
            tunnel: w512 -> [_ w545]
            tunnel: w511 -> [_ w544]
            tunnel: [0.0 w540] -> w505
            frame False {
            }
            frame True {
              n179 = Index Array(array=w545, index=w544) -> (element=w543:cluster{string[]})
              n180 = Unbundle(w543) -> (w542:string[])
              n181 = Fract/Exp String To Number(string=w542) -> (number=w541:dbl[])  [unwired: 4 out]
              n182 = Array Max & Min(array=w541) -> (max value=w540:dbl)  [unwired: 3 out]
            }
          }
          n183 = Array Max & Min(array=w523) -> (max value=w503:dbl, min value=w501:dbl)  [unwired: 2 out]
          n184 = Array Max & Min(array=w522) -> (max value=w509:dbl, min value=w507:dbl)  [unwired: 2 out]
          n185 = case shown="True" w510 {
            tunnel: w509 -> [w531 w538]
            tunnel: [w530 w538] -> w508
            tunnel: w507 -> [w529 w537]
            tunnel: [w528 w537] -> w506
            tunnel: w505 -> [w527 w536]
            tunnel: [w526 w532] -> w504
            tunnel: w503 -> [w526 w535]
            tunnel: [w525 w533] -> w502
            tunnel: w501 -> [w525 w534]
            frame False {
              n186 = Subtract(x=w529, y=w527) -> (x-y=w528:dbl)
              n187 = Add(x=w531, y=w527) -> (x+y=w530:dbl)
            }
            frame True {
              n188 = Add(x=w535, y=w536) -> (x+y=w532:dbl)
              n189 = Subtract(x=w534, y=w536) -> (x-y=w533:dbl)
            }
          }
          n190 = case shown="1, Default" w511 {
            tunnel: [w549 w563] -> w521
            tunnel: w504 -> [w549 w562]
            tunnel: w502 -> [w548 w559]
            tunnel: [w548 w558] -> w520
            tunnel: [w547 w551] -> w519
            tunnel: w508 -> [w547 w554]
            tunnel: [w546 w550] -> w518
            tunnel: w506 -> [w546 w552]
            tunnel: w517 -> [_ w564]
            tunnel: w516 -> [_ w561]
            tunnel: w515 -> [_ w555]
            tunnel: w514 -> [_ w553]
            frame 0 {
            }
            frame 1, Default {
              n191 = Greater?(x=w555, y=w554) -> (0:w556:bool)
              n192 = Greater?(x=w564, y=w562) -> (0:w565:bool)
              n193 = Less?(x=w553, y=w552) -> (x < y?=w557:bool)
              n194 = Less?(x=w561, y=w559) -> (x < y?=w560:bool)
              n195 = Select(t=w555, s=w556, f=w554) -> (s? t:f=w551:dbl)
              n196 = Select(t=w553, s=w557, f=w552) -> (s? t:f=w550:dbl)
              n197 = Select(t=w564, s=w565, f=w562) -> (s? t:f=w563:dbl)
              n198 = Select(t=w561, s=w560, f=w559) -> (s? t:f=w558:dbl)
            }
          }
        }
        n199 = Subtract(x=w492, y=w493) -> (x-y=w494:dbl)
        n200 = Subtract(x=w487, y=w486) -> (x-y=w489:dbl)
        n201 = Multiply(x=w494, y=0.1) -> (x*y=w491:dbl)
        n202 = Multiply(x=w489, y=0.1) -> (x*y=w490:dbl)
        n203 = Add(x=w492, y=w491) -> (x+y=w479:dbl)
        n204 = Subtract(x=w493, y=w491) -> (x-y=w476:dbl)
        n205 = Add(x=w487, y=w490) -> (x+y=w472:dbl)
        n206 = Subtract(x=w486, y=w490) -> (x-y=w481:dbl)
        n207 = Select(t=w479, s="Xmax", f="Xmax Val") -> (s? t:f=w477:dbl)
        n208 = Select(t=w476, s="Xmin", f="Xmin Val") -> (s? t:f=w484:dbl)
        n209 = Select(t=w472, s="Ymax", f="Ymax Val") -> (s? t:f=w470:dbl)
        n210 = Select(t=w481, s="Ymin", f="Ymin Val") -> (s? t:f=w485:dbl)
        n211 = property on="XY Graph" class="XYGraph (strict)"("X Scale.Range:Maximum"=w477, "X Scale.Range:Minimum"=w484, "Y Scale.Range:Maximum"=w470, "Y Scale.Range:Minimum"=w485) -> ()  [unwired: 2 in, 2 out]
      }
      frame "Sort out plot title" {
        n212 = local read "Summarise"() -> (w579:u16)
        n213 = case shown="1, Default" "Plot Title" {
          selector: "Plot Title" -> [_ w597]
          tunnel: [w596 w603] -> w574
          tunnel: "Plot Title" -> [w596 w602]
          tunnel: w575 -> [_ w606]
          tunnel: w579 -> [_ w600]
          frame 0 {
          }
          frame 1, Default {
            n214 = Decrement(x=w597) -> (x-1=w605:u16)
            n215 = Add(x=w600, y=u16 2) -> (x+y=w599:u16)
            n216 = Index Array(array=w606, index (row)=w605, index (col)=w599) -> (element=w609:string)
            n217 = Empty String/Path?(string/path=w602) -> (empty?=w604:bool)
            n218 = call "Fast_string_Replace.vi"("Replace match with:"="~ ", "Input String"=w609, "regular expression"=":") -> ("Output String"=w608:string)  [unwired: 2 out]
            n219 = call <vilib>:"Trim Whitespace.vi"("string"=w608) -> ("trimmed string"=w607:string)  [unwired: 1 in]
            n220 = call "Fast_string_Replace.vi"("Replace match with:"="~", "Input String"=w607, "regular expression"="_") -> ("Output String"=w598:string)  [unwired: 2 out]
            n221 = case shown="False" w604 {
              tunnel: [w615 w618] -> w603
              tunnel: w598 -> [w617 w618]
              tunnel: w602 -> [w616 _]
              frame False {
                n222 = Concatenate Strings(w616, " " ("string"), w617) -> (w615:string)
              }
              frame True {
              }
            }
          }
        }
        n223 = case shown="False" "Show Labels?" {
          tunnel: w575 -> [w591 _]
          tunnel: w574 -> [w594 w595]
          tunnel: [w592 w595] -> w573
          frame False {
            n224 = local read "Added labels"() -> (w593:i32[])
            n225 = Concatenate Strings(w594, "         " ("string")) -> (w590:string)
            n226 = call "DistillTitle.vi"("Plot Summary in"=w591, "Show Channels with range of Values?"=FALSE, "Indices to include in Page Title"=w593, "String in"=w590) -> ("String out"=w592:string)  [unwired: 6 in, 1 out]
          }
          frame True {
          }
        }
        "Final Title" <- w573
        n227 = Current VI's Path() -> (path=w571:path)
        n228 = call "Running_as_top_level.vi"("Vi path name"=w571) -> ("Top Level"=w569:bool)  [unwired: 1 out]
        n229 = case shown="True" w569 {
          tunnel: [w583 w586] -> w568
          tunnel: w567 -> [w583 _]
          tunnel: ["Get Filename" ("t") "Create plot directory"] -> w566
          frame False {
          }
          frame True {
            n230 = local read "Path"() -> (w585:path)
            n231 = Strip Path(path=w585) -> (name=w584:string)  [unwired: 1 out]
            n232 = Build Path(base path=w585, name or relative path=w584) -> (appended path=w586:path)
          }
        }
      }
      frame "Get Filename" {
        n233 = local read "Final Title"() -> (w622:string)
        n234 = case shown="\"% change\"" w624 {
          tunnel: ["" "Per_" "Spec_" "N_Spec_"] -> w623
          frame "None" {
          }
          frame "% change" {
          }
          frame "Spectrum" {
          }
          frame "Norm Spec" {
          }
        }
        n235 = Concatenate Strings(w623, w622) -> (w619:string)
        n236 = String Length(string=w622) -> (length=w621:i32)
        n237 = case shown="0" w621 {
          tunnel: [w639 w640] -> w620
          tunnel: w619 -> [w639 w642]
          frame 0 {
          }
          frame 1, Default {
            n238 = Concatenate Strings(w642, "_") -> (w640:string)
          }
        }
        n239 = call "Auto_filename.vi"("Filename Max length"="Filename Max length", "Prefix"=w620) -> ("Filename"=w626:string)
        n240 = Build Path(base path=w633, name or relative path=w626) -> (appended path=w630:path)
        n241 = File/Directory Info(path=w630) -> (error out=w631:errorcluster)  [unwired: 1 in, 6 out]
        n242 = Build Path(base path=w630, name or relative path=w626) -> (appended path=w637:path)
        n243 = Unbundle By Name(w631) -> ("status"=w629:bool)
        n244 = Select(t="Create plot directory", s=w629, f="Find a unique name") -> (s? t:f=w636:string)
      }
      frame "Find a unique name" {
        n245 = call "FindUniqueName.vi"("Max Length"=27, "PathIn"=w649) -> ("UniquedPath"=w648:path)  [unwired: 9 in]
      }
      frame "Create plot directory" {
        n246 = Strip Path(path=w657) -> (stripped path=→"Path":path)  [unwired: 1 out]
        n247 = call "Create_directory_path.vi"("Path name"=w657) -> ("Path name Out"=w662:path)  [unwired: 1 in, 1 out]
        n248 = Select(t="Save data analysis file", s="Save data analysis file", f="Save .dat file") -> (s? t:f=w660:string)
      }
      frame "Save data analysis file" {
        n249 = stacked-sequence {
          seq-local: [w677 _ _] -> [_ _ w721]
          seq-local: [_ w693 _] -> [_ _ w719]
          tunnel: w675 -> [_ _ w732]
          tunnel: [_ _ TRUE ("Top Level")] -> w674
          tunnel: [_ _ "Save .dat file"] -> w673
          tunnel: w672 -> [w680 w695 _]
          tunnel: w671 -> [_ _ _]
          tunnel: w670 -> [_ _ _]
          tunnel: w666 -> [_ w696 _]
          tunnel: w668 -> [w684 _ _]
          tunnel: w667 -> [w683 _ _]
          frame #0 {
            n250 = case shown="\"Norm Spec\"" w684 {
              tunnel: w683 -> [w687 w691]
              tunnel: [w686 w690] -> w682
              tunnel: ["Wavelength::[mm]" "Wavelength::[mm]"] -> w681
              frame "Spectrum", Default {
                n251 = Concatenate Strings(w687, ":Spectral:Energy") -> (w686:string)
              }
              frame "Norm Spec" {
                n252 = Concatenate Strings(w691, ":Normalised Spectral:Energy") -> (w690:string)
              }
            }
            n253 = Index Array(array=w680, index (col)=0 ("disabled index (col)")) -> (element=w678:string[])  [unwired: 1 in]
            n254 = Build Array (concatenate)(w681, w682, w678) -> (w677:string[])
          }
          frame #1 {
            n255 = for {
              tunnel: w696 -> [w707] mode=indexing
              tunnel: w695 -> [w704]
              shift-right: [w698] -> w693
              shift-left: string[][] [] -> [w697]
              i -> [w702]
              n256 = Unbundle(w707) -> ("Output"=w706:dbl[], "PercentageDifferenceArray"=w705:dbl[])
              n257 = Add(x=3 ("disabled index (col)"), y=w702) -> (x+y=w701:i32)
              n258 = Index Array(array=w704, index (col)=w701) -> (element=w700:string[])  [unwired: 1 in]
              n259 = for {
                tunnel: w706 -> [w713] mode=indexing
                tunnel: w705 -> [w712] mode=indexing
                tunnel: w700 -> [w709]
                tunnel: [w708] -> w699 mode=indexing
                n260 = call "Number_2_string.vi"("number"=w713) -> ("String"=w711:string)  [unwired: 1 in]
                n261 = call "Number_2_string.vi"("number"=w712) -> ("String"=w710:string)  [unwired: 1 in]
                n262 = Build Array (concatenate)(w711, w710, w709) -> (w708:string[])
              }
              n263 = Build Array (concatenate)(w697, w699) -> (w698:string[][])
            }
          }
          frame #2 {
            w728 = FALSE  # Append last row only
            w727 = FALSE  # exists?
            n264 = Strip Path(path=w732) -> (stripped path=w733:path, name=w735:string)
            n265 = Array Size(array=w719) -> (size(s)=w718:i32[])
            n266 = Concatenate Strings(w735, ".xls" ("string")) -> (w734:string)
            n267 = Index Array(array=w718, index=0) -> (element=w716:i32)
            n268 = Build Path(base path=w733, name or relative path=w734) -> (appended path=w722:path)
            n269 = Initialize Array("", w716) -> (w715:string[])
            n270 = Build Array (concatenate)(w715, w719) -> (w720:string[][])
            n271 = Initialize Array("", 10 ("Dimension Size")) -> (w726:string[])
            n272 = call "Asterisk_header.vi"("Channel names"=w726) -> ("Header string"=w723:string)
            n273 = call "Write_Ch_data_file.vi"("Append last row only"=w728, "Header string"=w723, "exists?"=w727, "Channel Values"=w720, "Channel names"=w721, "Filename"=w722) -> ()  [unwired: 1 in, 5 out]
          }
        }
      }
      frame "Save .dat file" {
        n274 = stacked-sequence {
          seq-local: [w750 _ _ _ _] -> [_ _ _ _ w870]
          seq-local: [_ w776 _ _ _] -> [_ _ _ _ w871]
          seq-local: [_ _ _ w809 _] -> [_ _ _ _ w872]
          seq-local: [_ _ w793 _ _] -> [_ _ _ w807 _]
          seq-local: [_ _ w785 _ _] -> [_ _ _ w804 _]
          seq-local: [_ _ w787 _ _] -> [_ _ _ w803 _]
          tunnel: w748 -> [_ _ _ _ w875]
          tunnel: [_ _ _ _ TRUE ("Top Level")] -> w747
          tunnel: [_ _ _ _ "Gnuplot script Start"] -> w746
          tunnel: w745 -> [w755 _ _ _ _]
          tunnel: w744 -> [_ w779 _ _ _]
          tunnel: w743 -> [_ w775 _ _ _]
          tunnel: w742 -> [_ _ _ w811 _]
          tunnel: w741 -> [_ _ _ w808 _]
          tunnel: w740 -> [_ w773 _ _ _]
          tunnel: [_ _ _ w806 _] -> w739
          tunnel: w738 -> [_ _ w791 _ _]
          tunnel: w737 -> [_ _ _ w805 _]
          tunnel: w736 -> [_ _ w788 _ _]
          frame #0 {
            n275 = Array Subset(array=w755, length (col)=3 ("length")) -> (w753:string[][])  [unwired: 3 in]
            n276 = Build Array("Column Name", "Numeric Tolerance", "Range of Values") -> (w759:string[])
            n277 = Build Array (concatenate)(w759, w753) -> (w751:string[][])
            n278 = for {
              shift-right: [w763] -> w750
              shift-left: "" -> [w760]
              tunnel: w751 -> [w764] mode=indexing
              n279 = for {
                shift-right: [w765] -> w762
                shift-left: w760 -> [w772]
                tunnel: w764 -> [w766] mode=indexing
                i -> [w771]
                n280 = Equal To 0?(x=w771) -> (x = 0?=w770:bool)
                n281 = Select(t="#", s=w770, f="\t") -> (s? t:f=w767:string)
                n282 = Concatenate Strings(w772, w767, w766) -> (w765:string)
              }
              n283 = Concatenate Strings(w762, "\n") -> (w763:string)
            }
          }
          frame #1 {
            w777 = "\n"
            n284 = case shown="\"% change\"" w773 {
              tunnel: w775 -> [w781 w783]
              tunnel: [w781 w782] -> w774
              frame "None", Default {
              }
              frame "% change" {
                n285 = Concatenate Strings(w783, " %" ("string")) -> (w782:string)
              }
            }
            n286 = Concatenate Strings(w777, w777, "#" ("string"), w779, "\t", w774, w777, w777) -> (w776:string)
          }
          frame #2 {
            n287 = global read "Results_plotter_Global.vi" "Precision"() -> (w790:string[])
            n288 = global read "Results_plotter_Global.vi" "Absisca"() -> (w789:i32)
            n289 = case shown="True" "Offset?" {
              tunnel: [0.0 w801] -> w794
              frame False {
              }
              frame True {
                n290 = property on="XY Graph" class="XYGraph (strict)"() -> ("Y Scale.Range:Maximum"=w800:dbl, "Y Scale.Range:Minimum"=w802:dbl)  [unwired: 2 in, 2 out]
                n291 = Subtract(x=w800, y=w802) -> (x-y=w801:dbl)
              }
            }
            "Profile offset" <- w794
            n292 = Index Array(array=w790, index=w789) -> (element=w786:string)
            n293 = case shown="False" w788 {
              tunnel: ["" w798] -> w787
              tunnel: w786 -> [w795 w798]
              tunnel: [w795 ""] -> w785
              frame False {
              }
              frame True {
              }
            }
            n294 = Multiply(x=w794, y=w791) -> (x*y=w793:dbl)
          }
          frame #3 {
            n295 = for {
              tunnel: w811 -> [w838] mode=indexing
              shift-right: [w837] -> w809
              shift-left: "" -> [w828]
              tunnel: w808 -> [w826] mode=indexing
              tunnel: w807 -> [w823]
              tunnel: [w829] -> w806 mode=indexing
              tunnel: w805 -> [w816] mode=indexing
              tunnel: w804 -> [w813]
              tunnel: w803 -> [w812]
              i -> [w833]
              w836 = "\n"
              n296 = Multiply(x=w823, y=w833) -> (x*y=w818:dbl)
              n297 = Unbundle(w838) -> ("Output"=w831:dbl[], "PercentageDifferenceArray"=w832:dbl[])
              n298 = Negate(x=w818) -> (-x=w817:dbl)
              n299 = call "Number_2_string.vi"("number"=w817) -> ("String"=w825:string)  [unwired: 1 in]
              n300 = Format Into String(format string="\\t%s\\tPlot offset", w825) -> (resulting string=w821:string)  [unwired: 2 in, 1 out]
              n301 = Equal To 0?(x=w818) -> (x = 0?=w822:bool)
              n302 = Select(t="", s=w822, f=w821) -> (s? t:f=w819:string)
              n303 = Unbundle(w816) -> (w815:string[])
              n304 = for {
                tunnel: w831 -> [w857] mode=indexing
                shift-right: [w846] -> w835
                shift-left: "" -> [w847]
                tunnel: w832 -> [w854] mode=indexing
                tunnel: w818 -> [w853]
                tunnel: [w852] -> w830 mode=indexing
                tunnel: w815 -> [w849]
                shift-right: [w845] -> _
                shift-left: string[] [] -> [w844]
                tunnel: w813 -> [w841]
                tunnel: w812 -> [w840]
                i -> [w850]
                w851 = "\t"
                n305 = Subtract(x=w854, y=w853) -> (x-y=w852:dbl)
                n306 = call "Number_2_string.vi"("precision"=w841, "number"=w857) -> ("String"=w856:string)
                n307 = call "Number_2_string.vi"("precision"=w840, "number"=w852) -> ("String"=w855:string)
                n308 = Index Array(array=w849, index=w850) -> (element=w848:string)
                n309 = Concatenate Strings(w856, w851, w855, w851, w848, "\n") -> (w843:string)
                n310 = Search 1D Array(1D array=w844, element=w843) -> (index of element=w842:i32)  [unwired: 1 in]
                n311 = case shown="-1" w842 {
                  tunnel: w847 -> [w859 w864]
                  tunnel: [w859 w863] -> w846
                  tunnel: w843 -> [_ w860]
                  tunnel: w844 -> [w858 w862]
                  tunnel: [w858 w861] -> w845
                  frame 0, Default {
                  }
                  frame -1 {
                    n312 = Concatenate Strings(w864, w860) -> (w863:string)
                    n313 = Build Array (concatenate)(w862, w860) -> (w861:string[])
                  }
                }
              }
              n314 = Bundle("Output"=w831, w830) -> (w829:cluster{"Output":dbl[], dbl[]})  [unwired: 1 out]
              n315 = Concatenate Strings(w828, "#", w826, w819, w836, w835, w836, w836) -> (w837:string)
            }
          }
          frame #4 {
            w867 = FALSE  # advisory dialog? (display:T)
            w868 = FALSE  # append to file? (new file:F)
            n316 = Strip Path(path=w875) -> (stripped path=w876:path, name=w878:string)
            n317 = Concatenate Strings(w870, w871, w872) -> (w869:string)
            n318 = Concatenate Strings(w878, ".dat" ("string")) -> (w877:string)
            n319 = Build Path(base path=w876, name or relative path=w877) -> (appended path=w866:path)
            n320 = call "Write_Characters_To_File.vi"("file path (dialog if empty)"=w866, "advisory dialog? (display:T)"=w867, "character string"=w869, "append to file? (new file:F)"=w868) -> ()  [unwired: 1 in, 4 out]
          }
        }
      }
      frame "Gnuplot script Start" {
        n321 = case shown="\"None\", Default" w899 {
          tunnel: w898 -> [w916 w919 w923 w927]
          tunnel: [w916 w918 w922 w926] -> w886
          tunnel: [w915 w917 "Wavelength [mm]" ("X Axis Name") "Wavelength [mm]" ("X Axis Name")] -> w885
          tunnel: w897 -> [w915 w917 _ _]
          frame "None", Default {
          }
          frame "% change" {
            n322 = Concatenate Strings(w919, " % change" ("string")) -> (w918:string)
          }
          frame "Spectrum" {
            n323 = Concatenate Strings(w923, " Spectral energy" ("string")) -> (w922:string)
          }
          frame "Norm Spec" {
            n324 = Concatenate Strings(w927, " Normalised Spectral Energy" ("string")) -> (w926:string)
          }
        }
        n325 = local read "Final Title"() -> (w887:string)
        n326 = case shown="\"Linear\", Default" w891 {
          tunnel: [w906 w908 "Calculate fit parameters"] -> w890
          tunnel: "Edit Legend names" -> [w906 w908 _]
          tunnel: [w905 w907 "set parametric\nset samples 1000\n"] -> w879
          tunnel: "" -> [w905 w907 _]
          frame "None" {
          }
          frame "Spline" {
          }
          frame "Linear", Default {
          }
        }
        n327 = call "setTerm.vi"() -> ("String out"=w884:string)  [unwired: 10 in, 1 out]
        n328 = call "TypesetInsideMathmode.vi"("DirtyString"=w885) -> ("Mathmode String"=w881:string)  [unwired: 8 in, 2 out]
        n329 = call "TypesetInsideMathmode.vi"("DirtyString"=w886) -> ("Mathmode String"=w880:string)  [unwired: 8 in, 2 out]
        n330 = call "TypesetInsideMathmode.vi"("DirtyString"=w887) -> ("Mathmode String"=w883:string)  [unwired: 8 in, 2 out]
        n331 = local read "Time format?"() -> (w892:bool)
        n332 = call "setTitle.vi"("Title"=w883, "String in"=w884) -> ("String out"=w882:string)  [unwired: 8 in, 1 out]
        n333 = Format Into String(format string="set xlabel '%s'\nset ylabel '%s'\nset size %s,%s\n%s", initial string=w882, w881, w880, "Graph width", "Graph Height", w879) -> (resulting string=w894:string)  [unwired: 1 in, 1 out]
        n334 = case shown="True" w892 {
          tunnel: w894 -> [w911 w913]
          tunnel: [w911 w912] -> w893
          frame False {
          }
          frame True {
            n335 = Concatenate Strings(w913, "\nset xdata time\nset timefmt \"%s\"\nset format  x \"%H:%M\\n%Y-%m-%d\"\n") -> (w912:string)
          }
        }
      }
      frame "Calculate fit parameters" {
        # "k=1;    # label 1\nlab=\"23 mA\";\neval( sprintf (\"set label %d %s\", k, lab))"
        n336 = Strip Path(path=w944) -> (name=w943:string)  [unwired: 1 out]
        n337 = Select(t="2:1", s=w933, f="1:2") -> (s? t:f=w934:string)
        n338 = for {
          tunnel: w946 -> [w962]
          tunnel: w943 -> [w960]
          shift-right: [w958] -> w931
          shift-left: w942 -> [w959]
          tunnel: "Auto Zp" -> [w957]
          tunnel: "Fixed Zp" -> [w956]
          tunnel: w934 -> [w955]
          tunnel: w933 -> [w954]
          tunnel: w932 -> [w953] mode=indexing
          tunnel: [w948] -> w929
          i -> [w961]
          n339 = Unbundle(w953) -> ("Output"=w951:dbl[], "PercentageDifferenceArray"=w949:dbl[])
          n340 = case shown="False" w954 {
            tunnel: [w964 w966] -> w952
            tunnel: w951 -> [w964 w965]
            tunnel: [w963 w965] -> w950
            tunnel: w949 -> [w963 w966]
            frame False {
            }
            frame True {
            }
          }
          n341 = case shown="\"Gauss Lat\"" w962 {
            tunnel: w961 -> [w976 w997 w1012 w1031 w1055 w1059 w1065 w1071 _]
            tunnel: w960 -> [w978 w998 w1006 w1036 w1056 w1060 w1066 w1072 _]
            tunnel: w959 -> [w986 w1001 w1021 w1046 w1054 w1062 w1068 w1074 w1076]
            tunnel: [w985 w988 w1020 w1045 w1053 w1061 w1067 w1073 w1076] -> w958
            tunnel: w957 -> [_ _ w1011 w1035 _ _ _ _ _]
            tunnel: w956 -> [_ _ w1008 w1032 _ _ _ _ _]
            tunnel: w955 -> [w968 w989 w1005 w1027 w1052 w1058 w1064 w1070 _]
            tunnel: w952 -> [w969 w990 w1004 w1029 _ _ _ _ _]
            tunnel: w950 -> [w970 w991 w1003 w1028 _ _ _ _ _]
            tunnel: [w967 w987 w1002 w1026 w1051 w1057 w1063 w1069 ""] -> w948
            frame "Gauss Lat" {
              w973 = 0.01  # A value of zero make gnuplot stop working
              w967 = "\nf%d(t) = cmax%d*exp(-((t-offset%d)**2)/(2*sig%d**2))\ncmax%d = %.2f; sig%d = %.2f; offset%d = %.2f           # initial guess for cmax and sig and offset\nfit f%d(t) \"%s.dat\" index %d using %s via cmax%d, sig%d, offset%d #this is a gaussian fit\n"
              n342 = Array Max & Min(array=w970) -> (max value=w980:dbl, max index (indices)=w977:i32)  [unwired: 2 out]
              n343 = Array Max & Min(array=w969) -> (max value=w984:dbl, min value=w983:dbl)  [unwired: 2 out]
              n344 = Index Array(array=w969, index=w977) -> (element=w972:dbl)
              n345 = Subtract(x=w984, y=w983) -> (x-y=w982:dbl)
              n346 = Divide(x=w982, y=6.0) -> (x/y=w979:dbl)
              n347 = Absolute Value(x=w972) -> (abs(x)=w974:dbl)
              n348 = Greater?(x=w974, y=w973) -> (0:w975:bool)
              n349 = Select(t=w972, s=w975, f=w973) -> (s? t:f=w971:dbl)
              n350 = Format Into String(format string=w967, initial string=w986, w976, w976, w976, w976, w976, w980, w976, w979, w976, w971, w976, w978, w976, w968, w976, w976, w976) -> (resulting string=w985:string)  [unwired: 1 in, 1 out]
            }
            frame "Guass glc" {
              w994 = 0.01 ("y")
              w987 = "\nf%d(t) = cmax%d*((t/xmax%d)**(-(1+m%d)*q%d)*exp(((1+m%d)/2)*(1-(t/xmax%d)**(-2*q%d))))\ncmax%d = %.2f; xmax%d = %.2f; m%d = 1;  q%d = 0.73         # initial guess for cmax and xmax q and m\nfit f%d(t) \"%s.dat\" index %d using %s via cmax%d, xmax%d, m%d, q%d  #this is a gaussian fit\n"
              n351 = Array Max & Min(array=w991) -> (max value=w1000:dbl, max index (indices)=w999:i32)  [unwired: 2 out]
              n352 = Index Array(array=w990, index=w999) -> (element=w993:dbl)
              n353 = Absolute Value(x=w993) -> (abs(x)=w995:dbl)
              n354 = Greater?(x=w995, y=w994) -> (0:w996:bool)
              n355 = Select(t=w993, s=w996, f=w994) -> (s? t:f=w992:dbl)
              n356 = Format Into String(format string=w987, initial string=w1001, w997, w997, w997, w997, w997, w997, w997, w997, w997, w1000, w997, w992, w997, w997, w997, w998, w997, w989, w997, w997, w997, w997) -> (resulting string=w988:string)  [unwired: 1 in, 1 out]
            }
            frame "Gauss vert" {
              (unwired) "f1(x) = cmax1*exp(-((x-offset1)**2)/(2*sig1**2))"
              w1002 = "\nf%d(t) = cmax%d*(exp(-((t-Zp%d)**2)/(2*sigZ%d**2))+exp(-((t+Zp%d)**2)/(2*sigZ%d**2)))\ncmax%d = %.2f; sigZ%d = %.2f; Zp%d = %.2f           # initial guess for cmax and sig and offset\nfit f%d(t) \"%s.dat\" index %d using %s via cmax%d, sigZ%d%s, Zp%d #this is a gaussian fit\n"
              n357 = Array Max & Min(array=w1003) -> (max value=w1015:dbl, max index (indices)=w1013:i32)  [unwired: 2 out]
              n358 = Array Max & Min(array=w1004) -> (max value=w1019:dbl, min value=w1018:dbl)  [unwired: 2 out]
              n359 = Index Array(array=w1004, index=w1013) -> (element=w1010:dbl)
              n360 = Subtract(x=w1019, y=w1018) -> (x-y=w1017:dbl)
              n361 = Divide(x=w1017, y=6.0) -> (x/y=w1014:dbl)
              n362 = case shown="False" w1011 {
                tunnel: [w1023 w1025] -> w1009
                tunnel: w1010 -> [_ w1025]
                tunnel: w1008 -> [w1023 _]
                tunnel: [" #" ""] -> w1007
                frame False {
                }
                frame True {
                }
              }
              n363 = Format Into String(format string=w1002, initial string=w1021, w1012, w1012, w1012, w1012, w1012, w1012, w1012, w1015, w1012, w1014, w1012, w1009, w1012, w1006, w1012, w1005, w1012, w1012, w1007, w1012) -> (resulting string=w1020:string)  [unwired: 1 in, 1 out]
            }
            frame "Gauss Vert with 2 sig" {
              w1026 = "\nf%d(t) = %s\ncmax%d = %.2f; sigZ_low%d = %.2f; sigZ_up%d = %.2f; Zp%d = %.2f           # initial guess for cmax and sig and offset\nfit f%d(t) \"%s.dat\" index %d using %s via cmax%d, sigZ_low%d, sigZ_up%d%s, Zp%d #this is a gaussian fit\n"
              n364 = Array Max & Min(array=w1028) -> (max value=w1038:dbl, max index (indices)=w1040:i32)  [unwired: 2 out]
              n365 = Array Max & Min(array=w1029) -> (max value=w1044:dbl, min value=w1043:dbl)  [unwired: 2 out]
              n366 = Index Array(array=w1029, index=w1040) -> (element=w1034:dbl)
              n367 = Subtract(x=w1044, y=w1043) -> (x-y=w1042:dbl)
              n368 = Divide(x=w1042, y=6.0) -> (x/y=w1037:dbl)
              n369 = call "Vert_Spread_2_Sig.vi"("Index"=w1031) -> ("resulting string"=w1039:string)
              n370 = case shown="False" w1035 {
                tunnel: [w1048 w1050] -> w1033
                tunnel: w1032 -> [w1048 _]
                tunnel: [" #" ""] -> w1030
                tunnel: w1034 -> [_ w1050]
                frame False {
                }
                frame True {
                }
              }
              n371 = Format Into String(format string=w1026, initial string=w1046, w1031, w1039, w1031, w1038, w1031, w1037, w1031, w1037, w1031, w1033, w1031, w1036, w1031, w1027, w1031, w1031, w1031, w1030, w1031) -> (resulting string=w1045:string)  [unwired: 1 in, 1 out]
            }
            frame "2nd Poly" {
              w1051 = "\nf%d(t) = c%d*t**2 + b%d*t + a%d\n#a%d = 40; b%d = 300; c%d = 1           # initial guess for cmax and sig and offset\nfit f%d(t) \"%s.dat\" index %d using %s via a%d, b%d, c%d #this is a 2nd order poly fit\n"
              n372 = Format Into String(format string=w1051, initial string=w1054, w1055, w1055, w1055, w1055, w1055, w1055, w1055, w1055, w1056, w1055, w1052, w1055, w1055, w1055) -> (resulting string=w1053:string)  [unwired: 1 in, 1 out]
            }
            frame "3rd Poly" {
              w1057 = "\nf%d(t) = d%d*t**3 +c%d*t**2 + b%d*t + a%d\n#a%d = 40; b%d = 300; c%d = 1; d%d = 1         # initial guess for cmax and sig and offset\nfit f%d(t) \"%s.dat\" index %d using %s via a%d, b%d, c%d, d%d #this is a 3rd order poly fit\n"
              n373 = Format Into String(format string=w1057, initial string=w1062, w1059, w1059, w1059, w1059, w1059, w1059, w1059, w1059, w1059, w1059, w1060, w1059, w1058, w1059, w1059, w1059, w1059) -> (resulting string=w1061:string)  [unwired: 1 in, 1 out]
            }
            frame "4th Poly" {
              w1063 = "\nf%d(t) = e%d*t**4 + d%d*t**3 +c%d*t**2 + b%d*t + a%d\n#a%d = 40; b%d = 300; c%d = 1; d%d = 1  e%d = 1       # initial guess for cmax and sig and offset\nfit f%d(t) \"%s.dat\" index %d using %s via a%d, b%d, c%d, d%d, e%d #this is a 3rd order poly fit\n"
              n374 = Format Into String(format string=w1063, initial string=w1068, w1065, w1065, w1065, w1065, w1065, w1065, w1065, w1065, w1065, w1065, w1065, w1065, w1066, w1065, w1064, w1065, w1065, w1065, w1065, w1065) -> (resulting string=w1067:string)  [unwired: 1 in, 1 out]
            }
            frame "Linear" {
              w1069 = "\nf%d(t) = b%d*t + c%d\n#a%d = 40; b%d = 300; c%d = 1           # initial guess for cmax and sig and offset\nfit f%d(t) \"%s.dat\" index %d using %s via b%d, c%d #this is a Linear fit\n"
              n375 = Format Into String(format string=w1069, initial string=w1074, w1071, w1071, w1071, w1071, w1071, w1071, w1071, w1072, w1071, w1070, w1071, w1071) -> (resulting string=w1073:string)  [unwired: 1 in, 1 out]
            }
            frame "Spline", Default {
            }
          }
        }
        n376 = call "ParsingFitFormulae.vi"("String"=w929) -> ("element"=w930:string)
        n377 = local write "Current Fit Formula"(w930) -> ()
        n378 = Concatenate Strings(w931, "save variables 'Coeff.txt'\n") -> (w940:string)
      }
      frame "Edit Legend names" {
        n379 = local read "Profile offset"() -> (w1085:dbl)
        n380 = for {
          tunnel: w1095 -> [w1110] mode=indexing
          tunnel: [w1109] -> w1094 mode=indexing
          tunnel: [w1108] -> w1090
          i -> [w1108]
          n381 = String Length(string=w1110) -> (length=w1113:i32)
          n382 = Subtract(x=w1113, y=2) -> (x-y=w1111:i32)
          n383 = String Subset(string=w1110, length (rest)=w1111) -> (substring=w1103:string)  [unwired: 1 out]
          n384 = Match Pattern(string=w1103, regular expression="=") -> (before substring=w1102:string, match substring=w1101:string, after substring=w1100:string)  [unwired: 2 out]
          n385 = call "Match_Pat_Case_In.vi"("String to match"="legend", "String"=w1102) -> ("offset past match"=w1105:i32)  [unwired: 1 in, 3 out]
          n386 = Greater Than 0?(x=w1105) -> (x > 0?=w1104:bool)
          n387 = case shown="False" w1104 {
            tunnel: [w1114 w1118] -> w1097
            tunnel: w1100 -> [w1115 w1118]
            tunnel: w1102 -> [w1117 _]
            tunnel: w1101 -> [w1116 _]
            frame False {
              n388 = Concatenate Strings(w1117, w1116, w1115) -> (w1114:string)
            }
            frame True {
            }
          }
          n389 = call "Fast_string_Replace.vi"("Replace match with:"=" ", "Input String"=w1097, "regular expression"="_") -> ("Output String"=w1096:string)  [unwired: 2 out]
          n390 = call "Text_for_latex.vi"("Input String"=w1096) -> ("Output String"=w1109:string)
        }
        n391 = Multiply(x=w1087, y=w1085) -> (x*y=w1089:dbl)
        n392 = Decrement(x=w1087) -> (x-1=w1086:dbl)
        n393 = Multiply(x=w1089, y=w1090) -> (x*y=w1084:dbl)
        n394 = Multiply(x=w1085, y=w1086) -> (x*y=w1083:dbl)
        n395 = Add(x=w1083, y=w1084) -> (x+y=→"Extra range":dbl)
        n396 = Equal To 0?(x="Legend Position") -> (x = 0?=w1080:bool)
        n397 = Select(t="Auto Legend Position", s=w1080, f="Specified Legend Position") -> (s? t:f=w1078:string)
      }
      frame "Auto Legend Position" {
        w1122 = T9 {"Appearance"={"layout"="horizontal", "text-sample order"="", "key order"="", "surroundingBox"="", "MaxRows"=0, "MaxCols"=0, "WidthAdjust"=0.0}, "Alignment"={"Horizontal"="center", "Vertical"="bottom"}, "Location"="", "\"At\" location"={"XcoordSys"="", "YcoordSys"="", "Xvalue"=0.0, "Yvalue"=0.0}}  # LegendProperties
        w1120 = "at"  # Location
        # "Don't know if any of this is really required-  maybe for offset plots.....?"
        n398 = property on="XY Graph" class="XYGraph (strict)"() -> ("X Scale.Range:Maximum"=w1131:dbl, "X Scale.Range:Minimum"=w1130:dbl, "Y Scale.Range:Minimum"=w1134:dbl, "Y Scale.Range:Maximum"=w1132:dbl)  [unwired: 2 in, 2 out]
        n399 = local read "Graph Height"() -> (w1142:string)
        n400 = case shown="True" w1137 {
          tunnel: w1131 -> [w1163 w1167]
          tunnel: w1130 -> [w1162 w1166]
          tunnel: [w1163 w1165] -> w1148
          tunnel: [w1162 w1164] -> w1144
          frame False {
          }
          frame True {
            n401 = Logarithm Base 10(1:w1167) -> (0:w1165:dbl)
            n402 = Logarithm Base 10(1:w1166) -> (0:w1164:dbl)
          }
        }
        n403 = case shown="True" w1140 {
          tunnel: w1132 -> [w1169 w1173]
          tunnel: w1134 -> [w1168 w1172]
          tunnel: [w1169 w1171] -> w1155
          tunnel: [w1168 w1170] -> w1133
          frame False {
          }
          frame True {
            n404 = Logarithm Base 10(1:w1172) -> (0:w1170:dbl)
            n405 = Logarithm Base 10(1:w1173) -> (0:w1171:dbl)
          }
        }
        n406 = local read "Extra range"() -> (w1135:dbl)
        n407 = Fract/Exp String To Number(string=w1142) -> (number=w1141:dbl)  [unwired: 4 out]
        n408 = Subtract(x=w1133, y=w1135) -> (x-y=w1154:dbl)
        n409 = Divide(x=0.35 ("y"), y=w1141) -> (x/y=w1153:dbl)
        n410 = Subtract(x=w1155, y=w1154) -> (x-y=w1151:dbl)
        n411 = Subtract(x=w1148, y=w1144) -> (x-y=w1147:dbl)
        n412 = Multiply(x=w1151, y=w1153) -> (x*y=w1157:dbl)
        n413 = Divide(x=w1151, y=10.0) -> (x/y=w1149:dbl)
        "Delta y" <- w1149
        n414 = Multiply(x=0.9 ("y"), y=w1147) -> (x*y=w1158:dbl)
        n415 = Multiply(x=w1147, y=-0.2 ("x")) -> (x*y=w1145:dbl)
        n416 = Subtract(x=w1154, y=w1157) -> (x-y=w1139:dbl)
        n417 = case shown="True" "Show legend?" {
          tunnel: w1139 -> [w1180 w1186]
          tunnel: [w1180 w1184] -> w1128
          tunnel: w1149 -> [_ w1187]
          frame False {
          }
          frame True {
            n418 = local read "No of Series"() -> (w1183:i32)
            n419 = Add(x=0.65, y=w1183) -> (x+y=w1182:dbl)
            n420 = Multiply(x=w1187, y=w1182) -> (x*y=w1185:dbl)
            n421 = Subtract(x=w1186, y=w1185) -> (x-y=w1184:dbl)
          }
        }
        "Y location" <- w1128
        n422 = Add(x=w1158, y=w1144) -> (x+y=w1138:dbl)
        n423 = Add(x=w1144, y=w1145) -> (x+y=→"X location":dbl)
        n424 = case shown="True" w1137 {
          tunnel: w1138 -> [w1174 w1176]
          tunnel: [w1174 w1175] -> w1126
          frame False {
          }
          frame True {
            n425 = Power Of 10(x=w1176) -> (10^x=w1175:dbl)
          }
        }
        n426 = case shown="True" w1140 {
          tunnel: w1139 -> [w1177 w1179]
          tunnel: [w1177 w1178] -> w1125
          frame False {
          }
          frame True {
            n427 = Power Of 10(x=w1179) -> (10^x=w1178:dbl)
          }
        }
        n428 = local read "Appearance"() -> (w1119:T6)
        n429 = Bundle By Name(cluster=w1122, "\"At\" location.Xvalue"=w1126, "\"At\" location.Yvalue"=w1125, "Location"=w1120, "Appearance"=w1119) -> (w1121:T9)
        n430 = call "setKey.vi"("LegendProperties"=w1121, "Set?"="Show legend?", "String in"=w1127) -> ("String out"=w1124:string)  [unwired: 7 in, 1 out]
      }
      frame "Specified Legend Position" {
        w1191 = T9 {"Appearance"={"layout"="horizontal", "text-sample order"="", "key order"="", "surroundingBox"="", "MaxRows"=0, "MaxCols"=0, "WidthAdjust"=0.0}, "Alignment"={"Horizontal"="center", "Vertical"="bottom"}, "Location"="", "\"At\" location"={"XcoordSys"="", "YcoordSys"="", "Xvalue"=0.0, "Yvalue"=0.0}}  # LegendProperties
        # "Not sure if stuff below is required, to provide \"Y location\"?"
        n431 = property on="XY Graph" class="XYGraph (strict)"() -> ("Y Scale.Range:Minimum"=w1201:dbl, "Y Scale.Range:Maximum"=w1199:dbl)  [unwired: 2 in, 2 out]
        n432 = local read "Graph Height"() -> (w1207:string)
        n433 = case shown="True" w1205 {
          tunnel: w1199 -> [w1220 w1224]
          tunnel: w1201 -> [w1219 w1223]
          tunnel: [w1220 w1222] -> w1213
          tunnel: [w1219 w1221] -> w1200
          frame False {
          }
          frame True {
            n434 = Logarithm Base 10(1:w1224) -> (0:w1222:dbl)
            n435 = Logarithm Base 10(1:w1223) -> (0:w1221:dbl)
          }
        }
        n436 = local read "Extra range"() -> (w1202:dbl)
        n437 = local read "Show legend?"() -> (w1192:bool)
        n438 = Fract/Exp String To Number(string=w1207) -> (number=w1206:dbl)  [unwired: 4 out]
        n439 = Subtract(x=w1200, y=w1202) -> (x-y=w1212:dbl)
        n440 = Divide(x=0.35 ("y"), y=w1206) -> (x/y=w1211:dbl)
        n441 = local read "Legend Position"() -> (w1195:u16)
        n442 = Subtract(x=w1213, y=w1212) -> (x-y=w1210:dbl)
        n443 = property on="Legend Position" class="Ring (strict)"() -> ("Strings []"=w1196:string[])  [unwired: 2 in, 2 out]
        n444 = Multiply(x=w1210, y=w1211) -> (x*y=w1215:dbl)
        n445 = Index Array(array=w1196, index=w1195) -> (element=w1189:string)
        n446 = Divide(x=w1210, y=10.0) -> (x/y=w1208:dbl)
        n447 = Subtract(x=w1212, y=w1215) -> (x-y=w1204:dbl)
        n448 = case shown="True" w1192 {
          tunnel: w1204 -> [w1225 w1231]
          tunnel: [w1225 w1229] -> w1197
          tunnel: w1208 -> [_ w1232]
          frame False {
          }
          frame True {
            n449 = local read "No of Series"() -> (w1228:i32)
            n450 = Add(x=0.65, y=w1228) -> (x+y=w1227:dbl)
            n451 = Multiply(x=w1232, y=w1227) -> (x*y=w1230:dbl)
            n452 = Subtract(x=w1231, y=w1230) -> (x-y=w1229:dbl)
          }
        }
        n453 = Bundle By Name(cluster=w1191, "Location"=w1189, "Appearance"="Appearance") -> (w1190:T9)
        n454 = local write "Y location"(w1197) -> ()
        n455 = call "setKey.vi"("LegendProperties"=w1190, "Set?"=w1192, "String in"=w1194) -> ("String out"=w1193:string)  [unwired: 7 in, 1 out]
      }
      frame "Labels?" {
        n456 = call "setAxisGrids.vi"("Minor Gridlines"="Minor Gridlines", "Major Gridlines"="Major Gridlines", "String in"=w1236) -> ("String out"=w1235:string)  [unwired: 7 in, 1 out]
        n457 = Array Size(array="Added labels") -> (size(s)=w1244:i32)
        n458 = local read "Show Labels?"() -> (w1238:bool)
        n459 = Greater Than 0?(x=w1244) -> (x > 0?=w1240:bool)
        n460 = And(x=w1238, y=w1240) -> (x .and. y?=w1239:bool)
        n461 = Select(t="Add Labels to plot", s=w1239, f="Set plot ranges" ("t")) -> (s? t:f=w1241:string)
      }
      frame "Add Labels to plot" {
        n462 = stacked-sequence {
          seq-local: [w1259 _] -> [_ w1304]
          tunnel: [_ w1305] -> w1256
          tunnel: w1255 -> [_ w1306]
          tunnel: [_ "Set plot ranges" ("t")] -> w1252
          tunnel: w1251 -> [w1262 _]
          tunnel: w1250 -> [_ w1301]
          tunnel: w1249 -> [_ w1299]
          frame #0 {
            n463 = local read "Added labels"() -> (w1264:i32[])
            n464 = Index Array(array=w1262, index (col)=0 ("disabled index (col)")) -> (element=w1263:string[])  [unwired: 1 in]
            n465 = for {
              tunnel: w1264 -> [w1289] mode=indexing
              tunnel: w1263 -> [w1294]
              tunnel: w1262 -> [w1293]
              tunnel: "Summarise" -> [w1292]
              shift-right: [w1280] -> w1259
              shift-left: string[] [] -> [w1281]
              n466 = Add(x=w1292, y=u16 2) -> (x+y=w1290:u16)
              n467 = Index Array(array=w1293, index (col)=w1290) -> (element=w1288:string[])  [unwired: 1 in]
              n468 = Index Array(array=w1294, index=w1289) -> (element=w1285:string)
              n469 = Index Array(array=w1288, index=w1289) -> (element=w1279:string)
              n470 = call "Fast_string_Replace.vi"("Replace match with:"=" ", "Input String"=w1285, "regular expression"=":") -> ("Output String"=w1284:string)  [unwired: 2 out]
              n471 = call <vilib>:"Trim Whitespace.vi"("string"=w1284) -> ("trimmed string"=w1283:string)  [unwired: 1 in]
              n472 = Match Pattern(string=w1279, regular expression="=") -> (offset past match=w1277:i32)  [unwired: 4 out]
              n473 = Less Than 0?(x=w1277) -> (x < 0?=w1276:bool)
              n474 = Select(t="%s = %s" ("format string"), s=w1276, f="%s %s" ("format string")) -> (s? t:f=w1273:string)
              n475 = Format Into String(format string=w1273, w1283, w1279) -> (resulting string=w1266:string)  [unwired: 2 in, 1 out]
              n476 = Match Pattern(string=w1266, regular expression=";") -> (offset past match=w1271:i32)  [unwired: 4 out]
              n477 = Match Pattern(string=w1266, regular expression=" to ") -> (offset past match=w1270:i32)  [unwired: 4 out]
              n478 = Less Than 0?(x=w1271) -> (x < 0?=w1268:bool)
              n479 = Less Than 0?(x=w1270) -> (x < 0?=w1269:bool)
              n480 = And(x=w1268, y=w1269) -> (x .and. y?=w1267:bool)
              n481 = case shown="False" w1267 {
                tunnel: w1281 -> [w1295 w1298]
                tunnel: [w1295 w1296] -> w1280
                tunnel: w1266 -> [_ w1297]
                frame False {
                }
                frame True {
                  n482 = Build Array (concatenate)(w1298, w1297) -> (w1296:string[])
                }
              }
            }
          }
          frame #1 {
            n483 = local read "Show legend?"() -> (w1300:bool)
            n484 = local read "X location"() -> (w1303:dbl)
            n485 = local read "Delta y"() -> (w1302:dbl)
            n486 = for {
              shift-right: [w1327] -> w1305
              shift-left: w1306 -> [w1328]
              tunnel: w1304 -> [w1324] mode=indexing
              tunnel: w1303 -> [w1310]
              tunnel: w1302 -> [w1329]
              tunnel: w1301 -> [w1323]
              tunnel: w1300 -> [w1312]
              tunnel: w1299 -> [w1308]
              i -> [w1330]
              n487 = call "Text_for_latex.vi"("Input String"=w1324) -> ("Output String"=w1318:string)
              n488 = case shown="False" w1308 {
                tunnel: w1310 -> [w1333 w1335]
                tunnel: [w1333 w1334] -> w1309
                frame False {
                }
                frame True {
                  n489 = Power Of 10(x=w1335) -> (10^x=w1334:dbl)
                }
              }
              n490 = String Length(string=w1318) -> (length=w1321:i32)
              n491 = Less?(x=w1321, y=20) -> (x < y?=w1313:bool)
              n492 = Compound Arithmetic op=AND(w1313, invert w1312) -> (w1311:bool)
              n493 = Increment(x=w1330) -> (x+1=w1331:i32)
              n494 = case shown="True" w1311 {
                tunnel: [w1336 w1338] -> w1319
                tunnel: w1318 -> [w1336 w1339]
                tunnel: "~~~~~~~~~~~" -> [_ w1337]
                frame False {
                }
                frame True {
                  n495 = Concatenate Strings(w1337, w1339) -> (w1338:string)
                }
              }
              n496 = Multiply(x=w1330, y=w1329) -> (x*y=w1325:dbl)
              n497 = local read "Y location"() -> (w1326:dbl)
              n498 = call "Number_2_string.vi"("number"=w1309) -> ("String"=w1316:string)  [unwired: 1 in]
              n499 = Subtract(x=w1326, y=w1325) -> (x-y=w1322:dbl)
              n500 = case shown="False" w1323 {
                tunnel: w1322 -> [w1340 w1342]
                tunnel: [w1340 w1341] -> w1315
                frame False {
                }
                frame True {
                  n501 = Power Of 10(x=w1342) -> (10^x=w1341:dbl)
                }
              }
              n502 = call "Number_2_string.vi"("number"=w1315) -> ("String"=w1314:string)  [unwired: 1 in]
              n503 = Format Into String(format string="set label %d '%s' at %s, %s\n", initial string=w1328, w1331, w1319, w1316, w1314) -> (resulting string=w1327:string)  [unwired: 1 in, 1 out]
            }
          }
        }
      }
      frame "Set plot ranges" {
        w1343 = ""
        (unwired) "set border"
        (unwired) "set nologscale  y"
        (unwired) "set logscale  y"
        w1345 = "#"
        w1347 = ""
        n504 = local read "Profile offset"() -> (w1370:dbl)
        n505 = property on="XY Graph" class="XYGraph (strict)"() -> ("X Scale.Range:Maximum"=w1380:dbl, "X Scale.Range:Minimum"=w1379:dbl, "Y Scale.Range:Maximum"=w1363:dbl, "Y Scale.Range:Minimum"=w1364:dbl)  [unwired: 2 in, 2 out]
        n506 = local read "Extra range"() -> (w1374:dbl)
        n507 = Decrement(x=w1369) -> (x-1=w1371:dbl)
        n508 = Multiply(x=w1370, y=w1371) -> (x*y=w1368:dbl)
        n509 = Add(x=w1368, y=w1363) -> (x+y=w1367:dbl)
        n510 = Subtract(x=w1364, y=w1374) -> (x-y=w1375:dbl)
        n511 = call "Number_2_string.vi"("number"=w1367) -> ("String"=w1352:string)  [unwired: 1 in]
        n512 = call "Gnuplot_offset_ytics.vi"("Separation"=w1369, "Mode"="Mode", "precision"="precision", "Legend"=w1372, "Max Plot Value"=w1363, "Profile offset"=w1370) -> ("concatenated string"=w1359:string)
        n513 = call "Number_2_string.vi"("number"=w1380) -> ("String"=w1354:string)  [unwired: 1 in]
        n514 = call "Number_2_string.vi"("number"=w1379) -> ("String"=w1355:string)  [unwired: 1 in]
        n515 = call "Number_2_string.vi"("number"=w1375) -> ("String"=w1353:string)  [unwired: 1 in]
        n516 = case shown="True" w1356 {
          tunnel: [w1392 w1394] -> w1350
          tunnel: w1355 -> [w1392 _]
          tunnel: [w1391 w1393] -> w1349
          tunnel: w1354 -> [w1391 _]
          tunnel: w1353 -> [_ w1394]
          tunnel: w1352 -> [_ w1393]
          frame False {
          }
          frame True {
          }
        }
        n517 = local read "Time format?"() -> (w1344:bool)
        n518 = Select(t="\nset logscale  x\n", s=w1361, f=w1347) -> (s? t:f=w1358:string)
        n519 = Select(t="\nset logscale  y\n", s=w1366, f=w1347) -> (s? t:f=w1360:string)
        n520 = case shown="\"Linear\", Default" w1351 {
          tunnel: w1350 -> [_ w1389]
          tunnel: w1349 -> [_ w1388]
          tunnel: ["" w1387] -> w1348
          frame "Spline" {
          }
          frame "Linear", Default {
            n521 = Format Into String(format string="set trange [%s : %s]", w1389, w1388) -> (resulting string=w1387:string)  [unwired: 2 in, 1 out]
          }
        }
        n522 = Select(t=w1343, s=w1344, f=w1345) -> (s? t:f=w1346:string)
        n523 = Format Into String(format string="%s set xrange [%s : %s] \n%s set autoscale x \n%s set yrange [%s : %s]\n%s set autoscale y\n", initial string=w1382, w1343, w1355, w1354, w1346, w1343, w1353, w1352, w1345) -> (resulting string=w1377:string)  [unwired: 1 in, 1 out]
        n524 = Concatenate Strings(w1377, w1348, w1358, w1360, w1359) -> (w1378:string)
      }
      frame "Plot Command" {
        n525 = case shown="True" w1404 {
          tunnel: ["yerrorbars" "xerrorbars"] -> w1403
          tunnel: ["" ", t"] -> w1402
          tunnel: ["t, " ""] -> w1401
          frame False {
          }
          frame True {
          }
        }
        n526 = Strip Path(path=w1416) -> (name=w1398:string)  [unwired: 1 out]
        n527 = Format Into String(format string="\nfile=\"%s.dat\"\n\nplot ", w1398) -> (resulting string=w1399:string)  [unwired: 2 in, 1 out]
        n528 = global read "Results_plotter_Global.vi" "Series Index"() -> (w1405:i32[])
        n529 = for {
          shift-right: [w1462] -> w1397
          shift-left: w1399 -> [w1463]
          tunnel: w1410 -> [w1461]
          tunnel: w1415 -> [w1456] mode=indexing
          tunnel: "Plot style" -> [w1457]
          tunnel: w1408 -> [w1444]
          tunnel: w1407 -> [w1455] mode=indexing
          tunnel: "plot error bars?" -> [w1451]
          tunnel: w1403 -> [w1435]
          tunnel: w1405 -> [w1428] mode=indexing
          tunnel: w1402 -> [w1431]
          tunnel: w1401 -> [w1430]
          tunnel: "Fit Line Width" -> [w1424]
          i -> [w1432]
          n530 = Index Array(array=w1457, index=w1428) -> (element=w1439:u16)
          n531 = Quotient & Remainder(x=w1428, y=8) -> (x-y*floor(x/y)=w1443:i32)  [unwired: 1 out]
          n532 = call "Fast_string_Replace.vi"("Replace match with:"="", "Input String"=w1456, "regular expression"="[$]") -> ("Output String"=w1446:string)  [unwired: 2 out]
          n533 = case shown="2" w1439 {
            tunnel: ["points" ("format string") "lines" ("format string") "linespoints" ("format string")] -> w1436
            frame 0, Default {
            }
            frame 1 {
            }
            frame 2 {
            }
          }
          n534 = case shown="\"Spline\"" w1461 {
            tunnel: w1432 -> [_ w1474 w1481 w1488 w1495 w1503 w1510 w1517 w1524 w1531]
            tunnel: ["" w1475 w1482 w1489 w1497 w1504 w1511 w1518 w1525 w1532] -> w1460
            tunnel: w1428 -> [_ w1473 w1480 w1486 w1494 w1502 w1509 w1516 w1523 w1530]
            tunnel: "Fit Line Type" -> [_ w1472 w1479 w1487 w1493 w1501 w1508 w1515 w1522 w1529]
            tunnel: w1431 -> [_ _ w1477 w1485 w1491 w1499 w1506 w1513 w1520 w1527]
            tunnel: w1430 -> [_ _ w1478 w1484 w1492 w1500 w1507 w1514 w1521 w1528]
            tunnel: w1424 -> [_ w1471 _ _ _ _ _ _ _ _]
            frame "None", Default {
            }
            frame "Spline" {
              n535 = Format Into String(format string="file index %d using 1:2 axes x1y1 title'' linecolor %d lw %d linetype %d  smooth csplines, ", w1474, w1473, w1471, w1472) -> (resulting string=w1475:string)  [unwired: 2 in, 1 out]
            }
            frame "Gauss Lat" {
              n536 = Format Into String(format string="%s cmax%d*exp(-((t-offset%d)**2)/(2*sig%d**2))%s  linecolor %d linetype %d title '', ", w1478, w1481, w1481, w1481, w1477, w1480, w1479) -> (resulting string=w1482:string)  [unwired: 2 in, 1 out]
            }
            frame "Gauss vert" {
              n537 = Format Into String(format string="%s cmax%d*(exp(-((t-Zp%d)**2)/(2*sigZ%d**2))+exp(-((t+Zp%d)**2)/(2*sigZ%d**2)))%s linecolor %d linetype %d title '', ", w1484, w1488, w1488, w1488, w1488, w1488, w1485, w1486, w1487) -> (resulting string=w1489:string)  [unwired: 2 in, 1 out]
            }
            frame "Gauss Vert with 2 sig" {
              n538 = call "Vert_Spread_2_Sig.vi"("Index"=w1495) -> ("resulting string"=w1496:string)
              n539 = Format Into String(format string="%s %s%s  linecolor %d linetype %d title '', ", w1492, w1496, w1491, w1494, w1493) -> (resulting string=w1497:string)  [unwired: 2 in, 1 out]
            }
            frame "Guass glc" {
              n540 = Format Into String(format string="%s cmax%d*((t/xmax%d)**(-(1+m%d)*q%d)*exp(((1+m%d)/2)*(1-(t/xmax%d)**(-2*q%d))))%s  linecolor %d linetype %d title '', ", w1500, w1503, w1503, w1503, w1503, w1503, w1503, w1503, w1499, w1502, w1501) -> (resulting string=w1504:string)  [unwired: 2 in, 1 out]
            }
            frame "2nd Poly" {
              n541 = Format Into String(format string="%s c%d*t**2 + b%d*t + a%d%s  linecolor %d linetype %d title 'fit%d', ", w1507, w1510, w1510, w1510, w1506, w1509, w1508, w1510) -> (resulting string=w1511:string)  [unwired: 2 in, 1 out]
            }
            frame "3rd Poly" {
              n542 = Format Into String(format string="%s d%d*t**3  + c%d*t**2 + b%d*t + a%d %s linecolor %d linetype %d title 'fit%d', ", w1514, w1517, w1517, w1517, w1517, w1513, w1516, w1515, w1517) -> (resulting string=w1518:string)  [unwired: 2 in, 1 out]
            }
            frame "4th Poly" {
              n543 = Format Into String(format string="%s e%d*t**4 + d%d*t**3  + c%d*t**2 + b%d*t + a%d%s  linecolor %d linetype %d title 'fit%d', ", w1521, w1524, w1524, w1524, w1524, w1524, w1520, w1523, w1522, w1524) -> (resulting string=w1525:string)  [unwired: 2 in, 1 out]
            }
            frame "Linear" {
              n544 = Format Into String(format string="%s b%d*t + c%d%s  linecolor %d linetype %d title 'fit%d', ", w1528, w1531, w1531, w1527, w1530, w1529, w1531) -> (resulting string=w1532:string)  [unwired: 2 in, 1 out]
            }
          }
          n545 = Index Array(array=w1444, index=w1443) -> (element=w1426:i32)
          n546 = case shown="True" "Black and white?" {
            tunnel: w1428 -> [w1465 _]
            tunnel: [w1465 0] -> w1427
            frame False {
            }
            frame True {
            }
          }
          n547 = Unbundle(w1455) -> (w1454:string[])
          n548 = Array Size(array=w1454) -> (size(s)=w1453:i32)
          n549 = Greater Than 0?(x=w1453) -> (x > 0?=w1452:bool)
          n550 = And(x=w1452, y=w1451) -> (x .and. y?=w1437:bool)
          n551 = Select(t=w1435, s=w1437, f=w1436) -> (s? t:f=w1434:string)
          n552 = Select(t=":3", s=w1437, f="") -> (s? t:f=w1447:string)
          n553 = Format Into String(format string="file index %d using 1:2%s axes x1y1 title '$%s$' with ", initial string=w1463, w1432, w1447, w1446) -> (resulting string=w1450:string)  [unwired: 1 in, 1 out]
          n554 = Format Into String(format string=" linecolor %d pointtype %d pointsize %.2f linetype %d, ", initial string=w1434, w1427, w1426, "Point Size", w1426) -> (resulting string=w1438:string)  [unwired: 1 in, 1 out]
          n555 = Concatenate Strings(w1450, w1438, w1460, "\\" ("string"), "\n") -> (w1462:string)
        }
        n556 = call "removeLastContinuation.vi"("String in"=w1397) -> ("String out"=w1396:string)  [unwired: 10 in]
        n557 = Concatenate Strings(w1414, w1396) -> (w1413:string)
      }
      frame "Write gnuplot file" {
        w1542 = FALSE  # append to file? (new file:F)
        w1543 = FALSE  # advisory dialog? (display:T)
        n558 = Strip Path(path=w1539) -> (stripped path=w1535:path)  [unwired: 1 out]
        n559 = Build Path(base path=w1535, name or relative path="gnuplot_script.txt") -> (appended path=w1544:path)
        n560 = call "gnuplot_legend.vi"("Plot style"=w1536, "Legend"=w1540) -> ()  [unwired: 1 out]
        n561 = call "Write_Characters_To_File.vi"("file path (dialog if empty)"=w1544, "advisory dialog? (display:T)"=w1543, "character string"=w1534, "append to file? (new file:F)"=w1542) -> ()  [unwired: 1 in, 4 out]
      }
      frame "Execute shell script" {
        n562 = call "Run_Gnuplot_Script.vi"("logfileName"=w1546, "workingDirectory"=w1547) -> ()  [unwired: 1 in]
      }
      frame "Has pdf been generated?" {
        n563 = Strip Path(path=w1560) -> (stripped path=w1562:path, name=w1564:string)
        n564 = Concatenate Strings(w1564, ".pdf" ("string")) -> (w1563:string)
        n565 = Build Path(base path=w1562, name or relative path=w1563) -> (appended path=w1559:path)
        n566 = call "Does_file_exist_(simple).vi"("Pathname"=w1559) -> ("exists?"=w1558:bool)
        n567 = case shown="False" w1558 {
          tunnel: ["Open Standard output file" ("f") "Input Fit Coefficients into results file?"] -> w1553
          frame False {
          }
          frame True {
          }
        }
        n568 = Select(t="Show Re-Run Gnuplot?", s="Show Re-Run Gnuplot?", f=w1553) -> (s? t:f=w1554:string)
      }
      frame "Show Re-Run Gnuplot?" {
        n569 = Strip Path(path=w1571) -> (stripped path=w1570:path)  [unwired: 1 out]
        n570 = call "Re_run_Gnuplot.vi"("Plot folder (dialog if empty)"=w1570) -> ()  [unwired: 1 in, 3 out]
      }
      frame "Input Fit Coefficients into results file?" {
        n571 = Greater?(x=w1581, y=T4."Spline" ("Fit type")) -> (0:w1580:bool)
        n572 = And(x="Put Coeff\nin Results file", y=w1580) -> (x .and. y?=w1578:bool)
      }
      frame "Read Fit Coefficients" {
        n573 = call "Fast_string_Replace.vi"("Replace match with:"="", "Input String"=w1588, "regular expression"=":") -> ("Output String"=w1587:string)  [unwired: 2 out]
        n574 = Strip Path(path=w1600) -> (stripped path=w1598:path)  [unwired: 1 out]
        n575 = Build Path(base path=w1598, name or relative path="Coeff.txt") -> (appended path=w1597:path)
        n576 = call "Read_File_Simple.vi"("Filename"=w1597) -> ("string"=w1595:string)  [unwired: 2 in, 7 out]
        n577 = for {
          tunnel: w1596 -> [w1624]
          tunnel: w1595 -> [w1623]
          tunnel: [w1613] -> w1594
          tunnel: w1593 -> [w1621] mode=indexing
          shift-right: [w1618] -> w1591
          shift-left: string[][] [] -> [w1619]
          tunnel: w1587 -> [w1605]
          i -> [w1615]
          n578 = case shown="\"Gauss Lat\"" w1624 {
            tunnel: w1615 -> [_ w1650 w1663 w1674 w1678 w1695 w1709]
            tunnel: [string[] [] w1646 w1659 w1671 w1686 w1701 w1713] -> w1612
            tunnel: [string[] [] w1642 w1655 w1668 w1683 w1698 w1712] -> w1622
            frame "None", Default {
            }
            frame "Gauss Lat" {
              n579 = Format Into String(format string="sig%d", w1650) -> (resulting string=w1648:string)  [unwired: 2 in, 1 out]
              n580 = Format Into String(format string="offset%d", w1650) -> (resulting string=w1647:string)  [unwired: 2 in, 1 out]
              n581 = Format Into String(format string="cmax%d", w1650) -> (resulting string=w1649:string)  [unwired: 2 in, 1 out]
              n582 = Build Array(":Max:Lat", ":Sig Y:", ":Yo:", ":FitFormula:Lat") -> (w1642:string[])
              n583 = Build Array(w1649, w1648, w1647) -> (w1646:string[])
            }
            frame "2nd Poly" {
              n584 = Format Into String(format string="b%d", w1663) -> (resulting string=w1661:string)  [unwired: 2 in, 1 out]
              n585 = Format Into String(format string="c%d", w1663) -> (resulting string=w1660:string)  [unwired: 2 in, 1 out]
              n586 = Format Into String(format string="a%d", w1663) -> (resulting string=w1662:string)  [unwired: 2 in, 1 out]
              n587 = Build Array(":Coeff:A", ":Coeff:B", ":Coeff:C", ":FitFormula:Poly2") -> (w1655:string[])
              n588 = Build Array(w1662, w1661, w1660) -> (w1659:string[])
            }
            frame "Linear" {
              n589 = Format Into String(format string="c%d", w1674) -> (resulting string=w1673:string)  [unwired: 2 in, 1 out]
              n590 = Format Into String(format string="b%d", w1674) -> (resulting string=w1672:string)  [unwired: 2 in, 1 out]
              n591 = Build Array(":Offset:A", ":Grad:B", ":FitFormula:Lin") -> (w1668:string[])
              n592 = Build Array(w1673, w1672) -> (w1671:string[])
            }
            frame "Gauss Vert with 2 sig" {
              n593 = Format Into String(format string="Zp%d", w1678) -> (resulting string=w1687:string)  [unwired: 2 in, 1 out]
              n594 = Format Into String(format string="cmax%d", w1678) -> (resulting string=w1689:string)  [unwired: 2 in, 1 out]
              n595 = Format Into String(format string="sigZ_low%d", w1678) -> (resulting string=w1679:string)  [unwired: 2 in, 1 out]
              n596 = Format Into String(format string="sigZ_up%d", w1678) -> (resulting string=w1688:string)  [unwired: 2 in, 1 out]
              n597 = Build Array(":Max:Vert", ":Sig Z:Upper", ":Sig Z:Lower", ":Zp:", ":FitFormula:Vert2sig") -> (w1683:string[])
              n598 = Build Array(w1689, w1688, w1679, w1687) -> (w1686:string[])
            }
            frame "Gauss vert" {
              n599 = Format Into String(format string="Zp%d", w1695) -> (resulting string=w1702:string)  [unwired: 2 in, 1 out]
              n600 = Format Into String(format string="cmax%d", w1695) -> (resulting string=w1703:string)  [unwired: 2 in, 1 out]
              n601 = Format Into String(format string="sigZ%d", w1695) -> (resulting string=w1694:string)  [unwired: 2 in, 1 out]
              n602 = Build Array(":Max:Vert", ":Sig Z:Upper", ":Sig Z:Lower", ":Zp:", ":FitFormula:Vert") -> (w1698:string[])
              n603 = Build Array(w1703, w1694, w1694, w1702) -> (w1701:string[])
            }
            frame "Guass glc" {
              n604 = Format Into String(format string="xmax%d", w1709) -> (resulting string=w1718:string)  [unwired: 2 in, 1 out]
              n605 = Format Into String(format string="m%d", w1709) -> (resulting string=w1717:string)  [unwired: 2 in, 1 out]
              n606 = Format Into String(format string="q%d", w1709) -> (resulting string=w1708:string)  [unwired: 2 in, 1 out]
              n607 = Format Into String(format string="cmax%d", w1709) -> (resulting string=w1719:string)  [unwired: 2 in, 1 out]
              n608 = Build Array(":MaxC:glc", ":MaxX:glc", ":m:glc", ":q:glc", ":FitFormula:glc") -> (w1712:string[])
              n609 = Build Array(w1719, w1718, w1717, w1708) -> (w1713:string[])
            }
          }
          n610 = global read "Results_plotter_Global.vi" "Full Ch Names"() -> (w1607:string[])
          n611 = global read "Results_plotter_Global.vi" "Absisca"() -> (w1608:i32)
          n612 = Index Array(array=w1607, index=w1608) -> (element=w1606:string)
          n613 = for {
            tunnel: w1605 -> [w1632]
            tunnel: w1622 -> [w1631] mode=indexing
            tunnel: [w1630] -> w1613 mode=indexing
            n614 = Concatenate Strings(w1632, w1631) -> (w1630:string)
          }
          n615 = Unbundle(w1621) -> ("Output"=w1616:dbl[])  [unwired: 1 out]
          n616 = Array Size(array=w1616) -> (size(s)=w1617:i32)
          n617 = for {
            tunnel: w1612 -> [w1638] mode=indexing
            tunnel: w1623 -> [w1635]
            tunnel: [w1633] -> w1611 mode=indexing
            n618 = Concatenate Strings(w1638, " = " ("string")) -> (w1636:string)
            n619 = Match Pattern(string=w1635, regular expression=w1636) -> (after substring=w1634:string)  [unwired: 4 out]
            n620 = call "Split_at_return.vi"("String"=w1634) -> ("before substring"=w1633:string)  [unwired: 1 in, 3 out]
          }
          n621 = call "ReformatFitFormula.vi"("Current Fit Formula"="Current Fit Formula", "Curve Fit Index"=w1615, "Variables"=w1612, "Channel Names"=w1613, "X Axis Full Ch Name"=w1606) -> ("Reformatted Current Fit Formula"=w1610:string)
          n622 = disable-structure shown="Enabled" {
            disable-tunnel: w1611 -> [w1627 w1628]
            disable-tunnel: w1610 -> [w1626 _]
            disable-tunnel: [w1625 w1628] -> w1609
            frame Enabled {
              n623 = Build Array (concatenate)(w1627, w1626) -> (w1625:string[])
            }
            frame Disabled {
            }
          }
          n624 = for {
            N: w1617 -> [_]
            tunnel: w1609 -> [w1629]
            tunnel: [w1629] -> w1620 mode=indexing
          }
          n625 = Build Array (concatenate)(w1619, w1620) -> (w1618:string[][])
        }
        n626 = global write "Results_plotter_Global.vi" "New Chs In"(w1594) -> ()
        n627 = global write "Results_plotter_Global.vi" "New Values In"(w1591) -> ()
      }
      frame "Open Standard output file" {
        n628 = Strip Path(path=w1727) -> (stripped path=w1724:path)  [unwired: 1 out]
        n629 = Format Into String(format string="open \"%s\"", w1725) -> (resulting string=w1723:string)  [unwired: 2 in, 1 out]
        n630 = call <vilib>:"System Exec.vi"("working directory"=w1724, "command line"=w1723) -> ()  [unwired: 4 in, 6 out]
      }
    }
  }
  "Tex Info String" <- w17
  "Saved Automatically?" <- FALSE
